vi "USBL_UA TRACKER for boat.vi"() -> ()   [LabVIEW 2017]
uses:
  <vilib>/Analysis/2dsp.llb/Decimate (single shot, DBL).vi
  <vilib>/DAQmx/read.llb/DAQmx Read (Analog 1D Wfm NChan NSamp).vi
  38e43d16-6990-4eb8-9d42-40b952a00b57.vi
  25bd1765-28c0-4687-a34a-e202199d80b9.vi
  7c68f900-8937-4c41-aeac-c7f4ae5d0ac2.vi
  eb8648f9-6bcc-41d4-a5ab-eca906629b06.vi
  bc7cbcab-f54e-4253-b3cf-52637ffe357f.vi
  b046c4bb-afd7-42e5-9fb2-1f2d57cd0f45.vi
  21d9bc29-df65-4687-956e-6793f94ae84a.vi
  72b5a707-0e99-42b5-ad5e-0d06ee7307bc.vi
  <vilib>/Array/Sort 2D Array - Pop Stack.vi
  <vilib>/Array/Sort 2D Array - Push Stack.vi
  38e43d16-6990-4eb8-9d42-40b952a00b57.vi/8e49d9bf-4fb6-4c6e-994e-0ca732c0081e.vi
  25bd1765-28c0-4687-a34a-e202199d80b9.vi/5aca4e67-a699-496d-8f3e-64a90ea83440.vi
  7c68f900-8937-4c41-aeac-c7f4ae5d0ac2.vi/c793c687-6163-4a47-8deb-c782a58a8736.vi
  eb8648f9-6bcc-41d4-a5ab-eca906629b06.vi/8c49c932-3fa2-411e-bf9f-69df11e121b8.vi
  bc7cbcab-f54e-4253-b3cf-52637ffe357f.vi/154f0d68-2825-48c0-8ee2-adf7998e7ff9.vi
  b046c4bb-afd7-42e5-9fb2-1f2d57cd0f45.vi/c2f5fb0a-7bab-41dc-aee0-b17c4b21b3df.vi
  21d9bc29-df65-4687-956e-6793f94ae84a.vi/e3f212c9-88b2-4250-9581-4cd035c99f0d.vi
  72b5a707-0e99-42b5-ad5e-0d06ee7307bc.vi/54bdf0c9-fde7-4a65-a34a-a18ed20cf916.vi
  <vilib>/Analysis/3filter.llb/FIR Filter (DBL).vi
  <vilib>/DAQmx/create/channels.llb/DAQmx Create Channel (AI-Voltage-Basic).vi
  <vilib>/DAQmx/configure/timing.llb/DAQmx Timing (Sample Clock).vi
  <vilib>/DAQmx/miscellaneous.llb/DAQmx Fill In Error Info.vi
  <vilib>/DAQmx/create/channels.llb/DAQmx Create Channel (CO-Pulse Generation-Frequency).vi
  <vilib>/DAQmx/configure/timing.llb/DAQmx Timing (Implicit).vi
  <vilib>/Analysis/NI_AALBase.lvlib
  <vilib>/Analysis/NI_AALPro.lvlib
  <vilib>/Analysis/NI_AAL_SigProc.lvlib
  <resource>/objmgr/daqmx.rc
  <vilib>/httpClient/LabVIEWHTTPClient.lvlib
panel:
  out "not detected number":i32
  out "DoA trial number":i32
  out "DoA":dbl
  out "Distance":dbl
  out "Display":bool
  out "DoA Estimation":bool
  out "Signal processing":bool
  in  "Map Format":string(combo)="roadmap"
  in  "Size X":dbl=450.0
  in  "Size Y":dbl=650.0
  in  "Zoom":sgl=16.0 format="%#.1g"
  in  "WebBrowser":refnum<k7>(container) caption="웹 브라우저"
  in  "Logitude":string="129.15510"
  in  "Latitude":string="35.17100"
  out "Scope":picture
  out "MovingAverage_Coefficient":dbl[](array[numeric])=[0.0004, 0.0004, 0.0004, 0.0004, 0.0004, 0.0004, 0.0004, 0.0004, 0.0004, 0.0004, 0.0004, 0.0004, 0.0004, 0.0004, 0.0004, 0.0004, 0.0004, 0.0004, 0.0004, 0.0004, 0.0004, 0.0004, 0.0004, 0.0004, 0.0004, 0.0004, 0.0004, 0.0004, 0.0004, 0.0004, 0.0004, 0.0004, 0.0004, 0.0004, 0.0004, 0.0004, 0.0004, 0.0004, 0.0004, 0.0004, 0.0004, 0.0004, 0.0004, 0.0004, 0.0004, 0.0004, 0.0004, 0.0004, 0.0004, 0.0004, 0.0004, 0.0004, 0.0004, 0.0004, 0.0004, 0.0004, 0.0004, 0.0004, 0.0004, 0.0004, 0.0004, 0.0004, 0.0004, 0.0004, 0.0004, 0.0004, 0.0004, 0.0004, 0.0004, 0.0004, 0.0004, 0.0004, 0.0004, 0.0004, 0.0004, 0.0004, 0.0004, 0.0004, 0.0004, 0.0004, 0.0004, 0.0004, 0.0004, 0.0004, 0.0004, 0.0004, 0.0004, 0.0004, 0.0004, 0.0004, 0.0004, 0.0004, 0.0004, 0.0004, 0.0004, 0.0004, 0.0004, 0.0004, 0.0004, 0.0004, 0.0004, 0.0004, 0.0004, 0.0004, 0.0004, 0.0004, 0.0004, 0.0004, 0.0004, 0.0004, 0.0004, 0.0004, 0.0004, 0.0004, 0.0004, 0.0004, 0.0004, 0.0004, 0.0004, 0.0004, 0.0004, 0.0004, 0.0004, 0.0004, 0.0004, 0.0004, 0.0004, 0.0004, 0.0004, 0.0004, 0.0004, 0.0004, 0.0004, 0.0004, 0.0004, 0.0004, 0.0004, 0.0004, 0.0004, 0.0004, 0.0004, 0.0004, 0.0004, 0.0004, 0.0004, 0.0004, 0.0004, 0.0004, 0.0004, 0.0004, 0.0004, 0.0004, 0.0004, 0.0004, 0.0004, 0.0004, 0.0004, 0.0004, 0.0004, 0.0004, 0.0004, 0.0004, 0.0004, 0.0004, 0.0004, 0.0004, 0.0004, 0.0004, 0.0004, 0.0004, 0.0004, 0.0004, 0.0004, 0.0004, 0.0004, 0.0004, 0.0004, 0.0004, 0.0004, 0.0004, 0.0004, 0.0004, 0.0004, 0.0004, 0.0004, 0.0004, 0.0004, 0.0004, 0.0004, 0.0004, 0.0004, 0.0004, 0.0004, 0.0004, 0.0004, 0.0004, 0.0004, 0.0004, 0.0004, 0.0004, 0.0004, 0.0004, 0.0004, 0.0004, 0.0004, 0.0004, 0.0004, 0.0004, 0.0004, 0.0004, 0.0004, 0.0004, 0.0004, 0.0004, 0.0004, 0.0004, 0.0004, 0.0004, 0.0004, 0.0004, 0.0004, 0.0004, 0.0004, 0.0004, 0.0004, 0.0004, 0.0004, 0.0004, 0.0004, 0.0004, 0.0004, 0.0004, 0.0004, 0.0004, 0.0004, 0.0004, 0.0004, 0.0004, 0.0004, 0.0004, 0.0004, 0.0004, 0.0004, 0.0004, 0.0004, 0.0004, 0.0004, 0.0004, 0.0004, 0.0004, 0.0004, 0.0004, 0.0004, 0.0004, 0.0004, 0.0004, 0.0004, 0.0004, 0.0004, 0.0004, 0.0004, 0.0004, 0.0004, 0.0004, 0.0004, 0.0004, 0.0004, 0.0004, 0.0004, 0.0004, 0.0004, 0.0004, 0.0004, 0.0004, 0.0004, 0.0004, 0.0004, 0.0004, 0.0004, 0.0004, 0.0004, 0.0004, 0.0004, 0.0004, 0.0004, 0.0004, 0.0004, 0.0004, 0.0004, 0.0004, 0.0004, 0.0004, 0.0004, 0.0004, 0.0004, 0.0004, 0.0004, 0.0004, 0.0004, 0.0004, 0.0004, 0.0004, 0.0004, 0.0004, 0.0004, 0.0004, 0.0004, 0.0004, 0.0004, 0.0004, 0.0004, 0.0004, 0.0004, 0.0004, 0.0004, 0.0004, 0.0004, 0.0004, 0.0004, 0.0004, 0.0004, 0.0004, 0.0004, 0.0004, 0.0004, 0.0004, 0.0004, 0.0004, 0.0004, 0.0004, 0.0004, 0.0004, 0.0004, 0.0004, 0.0004, 0.0004, 0.0004, 0.0004, 0.0004, 0.0004, 0.0004, 0.0004, 0.0004, 0.0004, 0.0004, 0.0004, 0.0004, 0.0004, 0.0004, 0.0004, 0.0004, 0.0004, 0.0004, 0.0004, 0.0004, 0.0004, 0.0004, 0.0004, 0.0004, 0.0004, 0.0004, 0.0004, 0.0004, 0.0004, 0.0004, 0.0004, 0.0004, 0.0004, 0.0004, 0.0004, 0.0004, 0.0004, 0.0004, 0.0004, 0.0004, 0.0004, 0.0004, 0.0004, 0.0004, 0.0004, 0.0004, 0.0004, 0.0004, 0.0004, 0.0004, 0.0004, 0.0004, 0.0004, 0.0004, 0.0004, 0.0004, 0.0004, 0.0004, 0.0004, 0.0004, 0.0004, 0.0004, 0.0004, 0.0004, 0.0004, 0.0004, 0.0004, 0.0004, 0.0004, 0.0004, 0.0004, 0.0004, 0.0004, 0.0004, 0.0004, 0.0004, 0.0004, 0.0004, 0.0004, 0.0004, 0.0004, 0.0004, 0.0004, 0.0004, 0.0004, 0.0004, 0.0004, 0.0004, 0.0004, 0.0004, 0.0004, 0.0004, 0.0004, 0.0004, 0.0004, 0.0004, 0.0004, 0.0004, 0.0004, 0.0004, 0.0004, 0.0004, 0.0004, 0.0004, 0.0004, 0.0004, 0.0004, 0.0004, 0.0004, 0.0004, 0.0004, 0.0004, 0.0004, 0.0004, 0.0004, 0.0004, 0.0004, 0.0004, 0.0004, 0.0004, 0.0004, 0.0004, 0.0004, 0.0004, 0.0004, 0.0004, 0.0004, 0.0004, 0.0004, 0.0004, 0.0004, 0.0004, 0.0004, 0.0004, 0.0004, 0.0004, 0.0004, 0.0004, 0.0004, 0.0004, 0.0004, 0.0004, 0.0004, 0.0004, 0.0004, 0.0004, 0.0004, 0.0004, 0.0004, 0.0004, 0.0004, 0.0004, 0.0004, 0.0004, 0.0004, 0.0004, 0.0004, 0.0004, 0.0004, 0.0004, 0.0004, 0.0004, 0.0004, 0.0004, 0.0004, 0.0004, 0.0004, 0.0004, 0.0004, 0.0004, 0.0004, 0.0004, 0.0004, 0.0004, 0.0004, 0.0004, 0.0004, 0.0004, 0.0004, 0.0004, 0.0004, 0.0004, 0.0004, 0.0004, 0.0004, 0.0004, 0.0004, 0.0004, 0.0004, 0.0004, 0.0004, 0.0004, 0.0004, 0.0004, 0.0004, 0.0004, 0.0004, 0.0004, 0.0004, 0.0004, 0.0004, 0.0004, 0.0004, 0.0004, 0.0004, 0.0004, 0.0004, 0.0004, 0.0004, 0.0004, 0.0004, 0.0004, 0.0004, 0.0004, 0.0004, 0.0004, 0.0004, 0.0004, 0.0004, 0.0004, 0.0004, 0.0004, 0.0004, 0.0004, 0.0004, 0.0004, 0.0004, 0.0004, 0.0004, 0.0004, 0.0004, 0.0004, 0.0004, 0.0004, 0.0004, 0.0004, 0.0004, 0.0004, 0.0004, 0.0004, 0.0004, 0.0004, 0.0004, 0.0004, 0.0004, 0.0004, 0.0004, 0.0004, 0.0004, 0.0004, 0.0004, 0.0004, 0.0004, 0.0004, 0.0004, 0.0004, 0.0004, 0.0004, 0.0004, 0.0004, 0.0004, 0.0004, 0.0004, 0.0004, 0.0004, 0.0004, 0.0004, 0.0004, 0.0004, 0.0004, 0.0004, 0.0004, 0.0004, 0.0004, 0.0004, 0.0004, 0.0004, 0.0004, 0.0004, 0.0004, 0.0004, 0.0004, 0.0004, 0.0004, 0.0004, 0.0004, 0.0004, 0.0004, 0.0004, 0.0004, 0.0004, 0.0004, 0.0004, 0.0004, 0.0004, 0.0004, 0.0004, 0.0004, 0.0004, 0.0004, 0.0004, 0.0004, 0.0004, 0.0004, 0.0004, 0.0004, 0.0004, 0.0004, 0.0004, 0.0004, 0.0004, 0.0004, 0.0004, 0.0004, 0.0004, 0.0004, 0.0004, 0.0004, 0.0004, 0.0004, 0.0004, 0.0004, 0.0004, 0.0004, 0.0004, 0.0004, 0.0004, 0.0004, 0.0004, 0.0004, 0.0004, 0.0004, 0.0004, 0.0004, 0.0004, 0.0004, 0.0004, 0.0004, 0.0004, 0.0004, 0.0004, 0.0004, 0.0004, 0.0004, 0.0004, 0.0004, 0.0004, 0.0004, 0.0004, 0.0004, 0.0004, 0.0004, 0.0004, 0.0004, 0.0004, 0.0004, 0.0004, 0.0004, 0.0004, 0.0004, 0.0004, 0.0004, 0.0004, 0.0004, 0.0004, 0.0004, 0.0004, 0.0004, 0.0004, 0.0004, 0.0004, 0.0004, 0.0004, 0.0004, 0.0004, 0.0004, 0.0004, 0.0004, 0.0004, 0.0004, 0.0004, 0.0004, 0.0004, 0.0004, 0.0004, 0.0004, 0.0004, 0.0004, 0.0004, 0.0004, 0.0004, 0.0004, 0.0004, 0.0004, 0.0004, 0.0004, 0.0004, 0.0004, 0.0004, 0.0004, 0.0004, 0.0004, 0.0004, 0.0004, 0.0004, 0.0004, 0.0004, 0.0004, 0.0004, 0.0004, 0.0004, 0.0004, 0.0004, 0.0004, 0.0004, 0.0004, 0.0004, 0.0004, 0.0004, 0.0004, 0.0004, 0.0004, 0.0004, 0.0004, 0.0004, 0.0004, 0.0004, 0.0004, 0.0004, 0.0004, 0.0004, 0.0004, 0.0004, 0.0004, 0.0004, 0.0004, 0.0004, 0.0004, 0.0004, 0.0004, 0.0004, 0.0004, 0.0004, 0.0004, 0.0004, 0.0004, 0.0004, 0.0004, 0.0004, 0.0004, 0.0004, 0.0004, 0.0004, 0.0004, 0.0004, 0.0004, 0.0004, 0.0004, 0.0004, 0.0004, 0.0004, 0.0004, 0.0004, 0.0004, 0.0004, 0.0004, 0.0004, 0.0004, 0.0004, 0.0004, 0.0004, 0.0004, 0.0004, 0.0004, 0.0004, 0.0004, 0.0004, 0.0004, 0.0004, 0.0004, 0.0004, 0.0004, 0.0004, 0.0004, 0.0004, 0.0004, 0.0004, 0.0004, 0.0004, 0.0004, 0.0004, 0.0004, 0.0004, 0.0004, 0.0004, 0.0004, 0.0004, 0.0004, 0.0004, 0.0004, 0.0004, 0.0004, 0.0004, 0.0004, 0.0004, 0.0004, 0.0004, 0.0004, 0.0004, 0.0004, 0.0004, 0.0004, 0.0004, 0.0004, 0.0004, 0.0004, 0.0004, 0.0004, 0.0004, 0.0004, 0.0004, 0.0004, 0.0004, 0.0004, 0.0004, 0.0004, 0.0004, 0.0004, 0.0004, 0.0004, 0.0004, 0.0004, 0.0004, 0.0004, 0.0004, 0.0004, 0.0004, 0.0004, 0.0004, 0.0004, 0.0004, 0.0004, 0.0004, 0.0004, 0.0004, 0.0004, 0.0004, 0.0004, 0.0004, 0.0004, 0.0004, 0.0004, 0.0004, 0.0004, 0.0004, 0.0004, 0.0004, 0.0004, 0.0004, 0.0004, 0.0004, 0.0004, 0.0004, 0.0004, 0.0004, 0.0004, 0.0004, 0.0004, 0.0004, 0.0004, 0.0004, 0.0004, 0.0004, 0.0004, 0.0004, 0.0004, 0.0004, 0.0004, 0.0004, 0.0004, 0.0004, 0.0004, 0.0004, 0.0004, 0.0004, 0.0004, 0.0004, 0.0004, 0.0004, 0.0004, 0.0004, 0.0004, 0.0004, 0.0004, 0.0004, 0.0004, 0.0004, 0.0004, 0.0004, 0.0004, 0.0004, 0.0004, 0.0004, 0.0004, 0.0004, 0.0004, 0.0004, 0.0004, 0.0004, 0.0004, 0.0004, 0.0004, 0.0004, 0.0004, 0.0004, 0.0004, 0.0004, 0.0004, 0.0004, 0.0004, 0.0004, 0.0004, 0.0004, 0.0004, 0.0004, 0.0004, 0.0004, 0.0004, 0.0004, 0.0004, 0.0004, 0.0004, 0.0004, 0.0004, 0.0004, 0.0004, 0.0004, 0.0004, 0.0004, 0.0004, 0.0004, 0.0004, 0.0004, 0.0004, 0.0004, 0.0004, 0.0004, 0.0004, 0.0004, 0.0004, 0.0004, 0.0004, 0.0004, 0.0004, 0.0004, 0.0004, 0.0004, 0.0004, 0.0004, 0.0004, 0.0004, 0.0004, 0.0004, 0.0004, 0.0004, 0.0004, 0.0004, 0.0004, 0.0004, 0.0004, 0.0004, 0.0004, 0.0004, 0.0004, 0.0004, 0.0004, 0.0004, 0.0004, 0.0004, 0.0004, 0.0004, 0.0004, 0.0004, 0.0004, 0.0004, 0.0004, 0.0004, 0.0004, 0.0004, 0.0004, 0.0004, 0.0004, 0.0004, 0.0004, 0.0004, 0.0004, 0.0004, 0.0004, 0.0004, 0.0004, 0.0004, 0.0004, 0.0004, 0.0004, 0.0004, 0.0004, 0.0004, 0.0004, 0.0004, 0.0004, 0.0004, 0.0004, 0.0004, 0.0004, 0.0004, 0.0004, 0.0004, 0.0004, 0.0004, 0.0004, 0.0004, 0.0004, 0.0004, 0.0004, 0.0004, 0.0004, 0.0004, 0.0004, 0.0004, 0.0004, 0.0004, 0.0004, 0.0004, 0.0004, 0.0004, 0.0004, 0.0004, 0.0004, 0.0004, 0.0004, 0.0004, 0.0004, 0.0004, 0.0004, 0.0004, 0.0004, 0.0004, 0.0004, 0.0004, 0.0004, 0.0004, 0.0004, 0.0004, 0.0004, 0.0004, 0.0004, 0.0004, 0.0004, 0.0004, 0.0004, 0.0004, 0.0004, 0.0004, 0.0004, 0.0004, 0.0004, 0.0004, 0.0004, 0.0004, 0.0004, 0.0004, 0.0004, 0.0004, 0.0004, 0.0004, 0.0004, 0.0004, 0.0004, 0.0004, 0.0004, 0.0004, 0.0004, 0.0004, 0.0004, 0.0004, 0.0004, 0.0004, 0.0004, 0.0004, 0.0004, 0.0004, 0.0004, 0.0004, 0.0004, 0.0004, 0.0004, 0.0004, 0.0004, 0.0004, 0.0004, 0.0004, 0.0004, 0.0004, 0.0004, 0.0004, 0.0004, 0.0004, 0.0004, 0.0004, 0.0004, 0.0004, 0.0004, 0.0004, 0.0004, 0.0004, 0.0004, 0.0004, 0.0004, 0.0004, 0.0004, 0.0004, 0.0004, 0.0004, 0.0004, 0.0004, 0.0004, 0.0004, 0.0004, 0.0004, 0.0004, 0.0004, 0.0004, 0.0004, 0.0004, 0.0004, 0.0004, 0.0004, 0.0004, 0.0004, 0.0004, 0.0004, 0.0004, 0.0004, 0.0004, 0.0004, 0.0004, 0.0004, 0.0004, 0.0004, 0.0004, 0.0004, 0.0004, 0.0004, 0.0004, 0.0004, 0.0004, 0.0004, 0.0004, 0.0004, 0.0004, 0.0004, 0.0004, 0.0004, 0.0004, 0.0004, 0.0004, 0.0004, 0.0004, 0.0004, 0.0004, 0.0004, 0.0004, 0.0004, 0.0004, 0.0004, 0.0004, 0.0004, 0.0004, 0.0004, 0.0004, 0.0004, 0.0004, 0.0004, 0.0004, 0.0004, 0.0004, 0.0004, 0.0004, 0.0004, 0.0004, 0.0004, 0.0004, 0.0004, 0.0004, 0.0004, 0.0004, 0.0004, 0.0004, 0.0004, 0.0004, 0.0004, 0.0004, 0.0004, 0.0004, 0.0004, 0.0004, 0.0004, 0.0004, 0.0004, 0.0004, 0.0004, 0.0004, 0.0004, 0.0004, 0.0004, 0.0004, 0.0004, 0.0004, 0.0004, 0.0004, 0.0004, 0.0004, 0.0004, 0.0004, 0.0004, 0.0004, 0.0004, 0.0004, 0.0004, 0.0004, 0.0004, 0.0004, 0.0004, 0.0004, 0.0004, 0.0004, 0.0004, 0.0004, 0.0004, 0.0004, 0.0004, 0.0004, 0.0004, 0.0004, 0.0004, 0.0004, 0.0004, 0.0004, 0.0004, 0.0004, 0.0004, 0.0004, 0.0004, 0.0004, 0.0004, 0.0004, 0.0004, 0.0004, 0.0004, 0.0004, 0.0004, 0.0004, 0.0004, 0.0004, 0.0004, 0.0004, 0.0004, 0.0004, 0.0004, 0.0004, 0.0004, 0.0004, 0.0004, 0.0004, 0.0004, 0.0004, 0.0004, 0.0004, 0.0004, 0.0004, 0.0004, 0.0004, 0.0004, 0.0004, 0.0004, 0.0004, 0.0004, 0.0004, 0.0004, 0.0004, 0.0004, 0.0004, 0.0004, 0.0004, 0.0004, 0.0004, 0.0004, 0.0004, 0.0004, 0.0004, 0.0004, 0.0004, 0.0004, 0.0004, 0.0004, 0.0004, 0.0004, 0.0004, 0.0004, 0.0004, 0.0004, 0.0004, 0.0004, 0.0004, 0.0004, 0.0004, 0.0004, 0.0004, 0.0004, 0.0004, 0.0004, 0.0004, 0.0004, 0.0004, 0.0004, 0.0004, 0.0004, 0.0004, 0.0004, 0.0004, 0.0004, 0.0004, 0.0004, 0.0004, 0.0004, 0.0004, 0.0004, 0.0004, 0.0004, 0.0004, 0.0004, 0.0004, 0.0004, 0.0004, 0.0004, 0.0004, 0.0004, 0.0004, 0.0004, 0.0004, 0.0004, 0.0004, 0.0004, 0.0004, 0.0004, 0.0004, 0.0004, 0.0004, 0.0004, 0.0004, 0.0004, 0.0004, 0.0004, 0.0004, 0.0004, 0.0004, 0.0004, 0.0004, 0.0004, 0.0004, 0.0004, 0.0004, 0.0004, 0.0004, 0.0004, 0.0004, 0.0004, 0.0004, 0.0004, 0.0004, 0.0004, 0.0004, 0.0004, 0.0004, 0.0004, 0.0004, 0.0004, 0.0004, 0.0004, 0.0004, 0.0004, 0.0004, 0.0004, 0.0004, 0.0004, 0.0004, 0.0004, 0.0004, 0.0004, 0.0004, 0.0004, 0.0004, 0.0004, 0.0004, 0.0004, 0.0004, 0.0004, 0.0004, 0.0004, 0.0004, 0.0004, 0.0004, 0.0004, 0.0004, 0.0004, 0.0004, 0.0004, 0.0004, 0.0004, 0.0004, 0.0004, 0.0004, 0.0004, 0.0004, 0.0004, 0.0004, 0.0004, 0.0004, 0.0004, 0.0004, 0.0004, 0.0004, 0.0004, 0.0004, 0.0004, 0.0004, 0.0004, 0.0004, 0.0004, 0.0004, 0.0004, 0.0004, 0.0004, 0.0004, 0.0004, 0.0004, 0.0004, 0.0004, 0.0004, 0.0004, 0.0004, 0.0004, 0.0004, 0.0004, 0.0004, 0.0004, 0.0004, 0.0004, 0.0004, 0.0004, 0.0004, 0.0004, 0.0004, 0.0004, 0.0004, 0.0004, 0.0004, 0.0004, 0.0004, 0.0004, 0.0004, 0.0004, 0.0004, 0.0004, 0.0004, 0.0004, 0.0004, 0.0004, 0.0004, 0.0004, 0.0004, 0.0004, 0.0004, 0.0004, 0.0004, 0.0004, 0.0004, 0.0004, 0.0004, 0.0004, 0.0004, 0.0004, 0.0004, 0.0004, 0.0004, 0.0004, 0.0004, 0.0004, 0.0004, 0.0004, 0.0004, 0.0004, 0.0004, 0.0004, 0.0004, 0.0004, 0.0004, 0.0004, 0.0004, 0.0004, 0.0004, 0.0004, 0.0004, 0.0004, 0.0004, 0.0004, 0.0004, 0.0004, 0.0004, 0.0004, 0.0004, 0.0004, 0.0004, 0.0004, 0.0004, 0.0004, 0.0004, 0.0004, 0.0004, 0.0004, 0.0004, 0.0004, 0.0004, 0.0004, 0.0004, 0.0004, 0.0004, 0.0004, 0.0004, 0.0004, 0.0004, 0.0004, 0.0004, 0.0004, 0.0004, 0.0004, 0.0004, 0.0004, 0.0004, 0.0004, 0.0004, 0.0004, 0.0004, 0.0004, 0.0004, 0.0004, 0.0004, 0.0004, 0.0004, 0.0004, 0.0004, 0.0004, 0.0004, 0.0004, 0.0004, 0.0004, 0.0004, 0.0004, 0.0004, 0.0004, 0.0004, 0.0004, 0.0004, 0.0004, 0.0004, 0.0004, 0.0004, 0.0004, 0.0004, 0.0004, 0.0004, 0.0004, 0.0004, 0.0004, 0.0004, 0.0004, 0.0004, 0.0004, 0.0004, 0.0004, 0.0004, 0.0004, 0.0004, 0.0004, 0.0004, 0.0004, 0.0004, 0.0004, 0.0004, 0.0004, 0.0004, 0.0004, 0.0004, 0.0004, 0.0004, 0.0004, 0.0004, 0.0004, 0.0004, 0.0004, 0.0004, 0.0004, 0.0004, 0.0004, 0.0004, 0.0004, 0.0004, 0.0004, 0.0004, 0.0004, 0.0004, 0.0004, 0.0004, 0.0004, 0.0004, 0.0004, 0.0004, 0.0004, 0.0004, 0.0004, 0.0004, 0.0004, 0.0004, 0.0004, 0.0004, 0.0004, 0.0004, 0.0004, 0.0004, 0.0004, 0.0004, 0.0004, 0.0004, 0.0004, 0.0004, 0.0004, 0.0004, 0.0004, 0.0004, 0.0004, 0.0004, 0.0004, 0.0004, 0.0004, 0.0004, 0.0004, 0.0004, 0.0004, 0.0004, 0.0004, 0.0004, 0.0004, 0.0004, 0.0004, 0.0004, 0.0004, 0.0004, 0.0004, 0.0004, 0.0004, 0.0004, 0.0004, 0.0004, 0.0004, 0.0004, 0.0004, 0.0004, 0.0004, 0.0004, 0.0004, 0.0004, 0.0004, 0.0004, 0.0004, 0.0004, 0.0004, 0.0004, 0.0004, 0.0004, 0.0004, 0.0004, 0.0004, 0.0004, 0.0004, 0.0004, 0.0004, 0.0004, 0.0004, 0.0004, 0.0004, 0.0004, 0.0004, 0.0004, 0.0004, 0.0004, 0.0004, 0.0004, 0.0004, 0.0004, 0.0004, 0.0004, 0.0004, 0.0004, 0.0004, 0.0004, 0.0004, 0.0004, 0.0004, 0.0004, 0.0004, 0.0004, 0.0004, 0.0004, 0.0004, 0.0004, 0.0004, 0.0004, 0.0004, 0.0004, 0.0004, 0.0004, 0.0004, 0.0004, 0.0004, 0.0004, 0.0004, 0.0004, 0.0004, 0.0004, 0.0004, 0.0004, 0.0004, 0.0004, 0.0004, 0.0004, 0.0004, 0.0004, 0.0004, 0.0004, 0.0004, 0.0004, 0.0004, 0.0004, 0.0004, 0.0004, 0.0004, 0.0004, 0.0004, 0.0004, 0.0004, 0.0004, 0.0004, 0.0004, 0.0004, 0.0004, 0.0004, 0.0004, 0.0004, 0.0004, 0.0004, 0.0004, 0.0004, 0.0004, 0.0004, 0.0004, 0.0004, 0.0004, 0.0004, 0.0004, 0.0004, 0.0004, 0.0004, 0.0004, 0.0004, 0.0004, 0.0004, 0.0004, 0.0004, 0.0004, 0.0004, 0.0004, 0.0004, 0.0004, 0.0004, 0.0004, 0.0004, 0.0004, 0.0004, 0.0004, 0.0004, 0.0004, 0.0004, 0.0004, 0.0004, 0.0004, 0.0004, 0.0004, 0.0004, 0.0004, 0.0004, 0.0004, 0.0004, 0.0004, 0.0004, 0.0004, 0.0004, 0.0004, 0.0004, 0.0004, 0.0004, 0.0004, 0.0004, 0.0004, 0.0004, 0.0004, 0.0004, 0.0004, 0.0004, 0.0004, 0.0004, 0.0004, 0.0004, 0.0004, 0.0004, 0.0004, 0.0004, 0.0004, 0.0004, 0.0004, 0.0004, 0.0004, 0.0004, 0.0004, 0.0004, 0.0004, 0.0004, 0.0004, 0.0004, 0.0004, 0.0004, 0.0004, 0.0004, 0.0004, 0.0004, 0.0004, 0.0004, 0.0004, 0.0004, 0.0004, 0.0004, 0.0004, 0.0004, 0.0004, 0.0004, 0.0004, 0.0004, 0.0004, 0.0004, 0.0004, 0.0004, 0.0004, 0.0004, 0.0004, 0.0004, 0.0004, 0.0004, 0.0004, 0.0004, 0.0004, 0.0004, 0.0004, 0.0004, 0.0004, 0.0004, 0.0004, 0.0004, 0.0004, 0.0004, 0.0004, 0.0004, 0.0004, 0.0004, 0.0004, 0.0004, 0.0004, 0.0004, 0.0004, 0.0004, 0.0004, 0.0004, 0.0004, 0.0004, 0.0004, 0.0004, 0.0004, 0.0004, 0.0004, 0.0004, 0.0004, 0.0004, 0.0004, 0.0004, 0.0004, 0.0004, 0.0004, 0.0004, 0.0004, 0.0004, 0.0004, 0.0004, 0.0004, 0.0004, 0.0004, 0.0004, 0.0004, 0.0004, 0.0004, 0.0004, 0.0004, 0.0004, 0.0004, 0.0004, 0.0004, 0.0004, 0.0004, 0.0004, 0.0004, 0.0004, 0.0004, 0.0004, 0.0004, 0.0004, 0.0004, 0.0004, 0.0004, 0.0004, 0.0004, 0.0004, 0.0004, 0.0004, 0.0004, 0.0004, 0.0004, 0.0004, 0.0004, 0.0004, 0.0004, 0.0004, 0.0004, 0.0004, 0.0004, 0.0004, 0.0004, 0.0004, 0.0004, 0.0004, 0.0004, 0.0004, 0.0004, 0.0004, 0.0004, 0.0004, 0.0004, 0.0004, 0.0004, 0.0004, 0.0004, 0.0004, 0.0004, 0.0004, 0.0004, 0.0004, 0.0004, 0.0004, 0.0004, 0.0004, 0.0004, 0.0004, 0.0004, 0.0004, 0.0004, 0.0004, 0.0004, 0.0004, 0.0004, 0.0004, 0.0004, 0.0004, 0.0004, 0.0004, 0.0004, 0.0004, 0.0004, 0.0004, 0.0004, 0.0004, 0.0004, 0.0004, 0.0004, 0.0004, 0.0004, 0.0004, 0.0004, 0.0004, 0.0004, 0.0004, 0.0004, 0.0004, 0.0004, 0.0004, 0.0004, 0.0004, 0.0004, 0.0004, 0.0004, 0.0004, 0.0004, 0.0004, 0.0004, 0.0004, 0.0004, 0.0004, 0.0004, 0.0004, 0.0004, 0.0004, 0.0004, 0.0004, 0.0004, 0.0004, 0.0004, 0.0004, 0.0004, 0.0004, 0.0004, 0.0004, 0.0004, 0.0004, 0.0004, 0.0004, 0.0004, 0.0004, 0.0004, 0.0004, 0.0004, 0.0004, 0.0004, 0.0004, 0.0004, 0.0004, 0.0004, 0.0004, 0.0004, 0.0004, 0.0004, 0.0004, 0.0004, 0.0004, 0.0004, 0.0004, 0.0004, 0.0004, 0.0004, 0.0004, 0.0004, 0.0004, 0.0004, 0.0004, 0.0004, 0.0004, 0.0004, 0.0004, 0.0004, 0.0004, 0.0004, 0.0004, 0.0004, 0.0004, 0.0004, 0.0004, 0.0004, 0.0004, 0.0004, 0.0004, 0.0004, 0.0004, 0.0004, 0.0004, 0.0004, 0.0004, 0.0004, 0.0004, 0.0004, 0.0004, 0.0004, 0.0004, 0.0004, 0.0004, 0.0004, 0.0004, 0.0004, 0.0004, 0.0004, 0.0004, 0.0004, 0.0004, 0.0004, 0.0004, 0.0004, 0.0004, 0.0004, 0.0004, 0.0004, 0.0004, 0.0004, 0.0004, 0.0004, 0.0004, 0.0004, 0.0004, 0.0004, 0.0004, 0.0004, 0.0004, 0.0004, 0.0004, 0.0004, 0.0004, 0.0004, 0.0004, 0.0004, 0.0004, 0.0004, 0.0004, 0.0004, 0.0004, 0.0004, 0.0004, 0.0004, 0.0004, 0.0004, 0.0004, 0.0004, 0.0004, 0.0004, 0.0004, 0.0004, 0.0004, 0.0004, 0.0004, 0.0004, 0.0004, 0.0004, 0.0004, 0.0004, 0.0004, 0.0004, 0.0004, 0.0004, 0.0004, 0.0004, 0.0004, 0.0004, 0.0004, 0.0004, 0.0004, 0.0004, 0.0004, 0.0004, 0.0004, 0.0004, 0.0004, 0.0004, 0.0004, 0.0004, 0.0004, 0.0004, 0.0004, 0.0004, 0.0004, 0.0004, 0.0004, 0.0004, 0.0004, 0.0004, 0.0004, 0.0004, 0.0004, 0.0004, 0.0004, 0.0004, 0.0004, 0.0004, 0.0004, 0.0004, 0.0004, 0.0004, 0.0004, 0.0004, 0.0004, 0.0004, 0.0004, 0.0004, 0.0004, 0.0004, 0.0004, 0.0004, 0.0004, 0.0004, 0.0004, 0.0004, 0.0004, 0.0004, 0.0004, 0.0004, 0.0004, 0.0004, 0.0004, 0.0004, 0.0004, 0.0004, 0.0004, 0.0004, 0.0004, 0.0004, 0.0004, 0.0004, 0.0004, 0.0004, 0.0004, 0.0004, 0.0004, 0.0004, 0.0004, 0.0004, 0.0004, 0.0004, 0.0004, 0.0004, 0.0004, 0.0004, 0.0004, 0.0004, 0.0004, 0.0004, 0.0004, 0.0004, 0.0004, 0.0004, 0.0004, 0.0004, 0.0004, 0.0004, 0.0004, 0.0004, 0.0004, 0.0004, 0.0004, 0.0004, 0.0004, 0.0004, 0.0004, 0.0004, 0.0004, 0.0004, 0.0004, 0.0004, 0.0004, 0.0004, 0.0004, 0.0004, 0.0004, 0.0004, 0.0004, 0.0004, 0.0004, 0.0004, 0.0004, 0.0004, 0.0004, 0.0004, 0.0004, 0.0004, 0.0004, 0.0004, 0.0004, 0.0004, 0.0004, 0.0004, 0.0004, 0.0004, 0.0004, 0.0004, 0.0004, 0.0004, 0.0004, 0.0004, 0.0004, 0.0004, 0.0004, 0.0004, 0.0004, 0.0004, 0.0004, 0.0004, 0.0004, 0.0004, 0.0004, 0.0004, 0.0004, 0.0004, 0.0004, 0.0004, 0.0004, 0.0004, 0.0004, 0.0004, 0.0004, 0.0004, 0.0004, 0.0004, 0.0004, 0.0004, 0.0004, 0.0004, 0.0004, 0.0004, 0.0004, 0.0004, 0.0004, 0.0004, 0.0004, 0.0004, 0.0004, 0.0004, 0.0004, 0.0004, 0.0004, 0.0004, 0.0004, 0.0004, 0.0004, 0.0004, 0.0004, 0.0004, 0.0004, 0.0004, 0.0004, 0.0004, 0.0004, 0.0004, 0.0004, 0.0004, 0.0004, 0.0004, 0.0004, 0.0004, 0.0004, 0.0004, 0.0004, 0.0004, 0.0004, 0.0004, 0.0004, 0.0004, 0.0004, 0.0004, 0.0004, 0.0004, 0.0004, 0.0004, 0.0004, 0.0004, 0.0004, 0.0004, 0.0004, 0.0004, 0.0004, 0.0004, 0.0004, 0.0004, 0.0004, 0.0004, 0.0004, 0.0004, 0.0004, 0.0004, 0.0004, 0.0004, 0.0004, 0.0004, 0.0004, 0.0004, 0.0004, 0.0004, 0.0004, 0.0004, 0.0004, 0.0004, 0.0004, 0.0004, 0.0004, 0.0004, 0.0004, 0.0004, 0.0004, 0.0004, 0.0004, 0.0004, 0.0004, 0.0004, 0.0004, 0.0004, 0.0004, 0.0004, 0.0004, 0.0004, 0.0004, 0.0004, 0.0004, 0.0004, 0.0004, 0.0004, 0.0004, 0.0004, 0.0004, 0.0004, 0.0004, 0.0004, 0.0004, 0.0004, 0.0004, 0.0004, 0.0004, 0.0004, 0.0004, 0.0004, 0.0004, 0.0004, 0.0004, 0.0004, 0.0004, 0.0004, 0.0004, 0.0004, 0.0004, 0.0004, 0.0004, 0.0004, 0.0004, 0.0004, 0.0004, 0.0004, 0.0004, 0.0004]
  out "Coefficient2_bit1":dbl[](array[numeric])
  out "Coefficient2_bit0":dbl[](array[numeric])
  in  "Start frequency(Hz) 2":dbl=30000.0 format="%#_6p"
  in  "Stop frequency(Hz) 2":dbl=34000.0 format="%#_6p"
  in  "Number of sample 2":i32=20000
  in  "Sampling freuqncy(Hz) 2":dbl=100000.0 format="%#_6p"
  out "Target code":dbl[](array[numeric])=[0.0, 1.0, 1.0, 1.0, 0.0, 0.0, 1.0, 0.0]
  in  "Number of pulse":i32=160
  in  "Output terminal":tag="/Dev4/PFI0"
  in  "Frequency(Hz)":dbl=32000.0 format="%.6f"
  in  "Cycle share":dbl=0.5 format="%.6f"
  in  "Counter":tag="Dev4/ctr0"
  out "Detect":bool
  in  "User number":i32=12
  in  "Start frequency(Hz)":dbl format="%#_6p"
  in  "Stop frequency(Hz)":dbl=4000.0 format="%#_6p"
  in  "Symbol length(sec)":dbl=0.128 format="%#_6p"
  in  "Number of sample":i32=38400
  in  "Sampling freuqncy(Hz)":dbl=192000.0 format="%#_6p"
  in  "Physical channel":tag="Dev4/ai0:7" caption="Physical Channel"
  in  "Device":tag="Dev4"
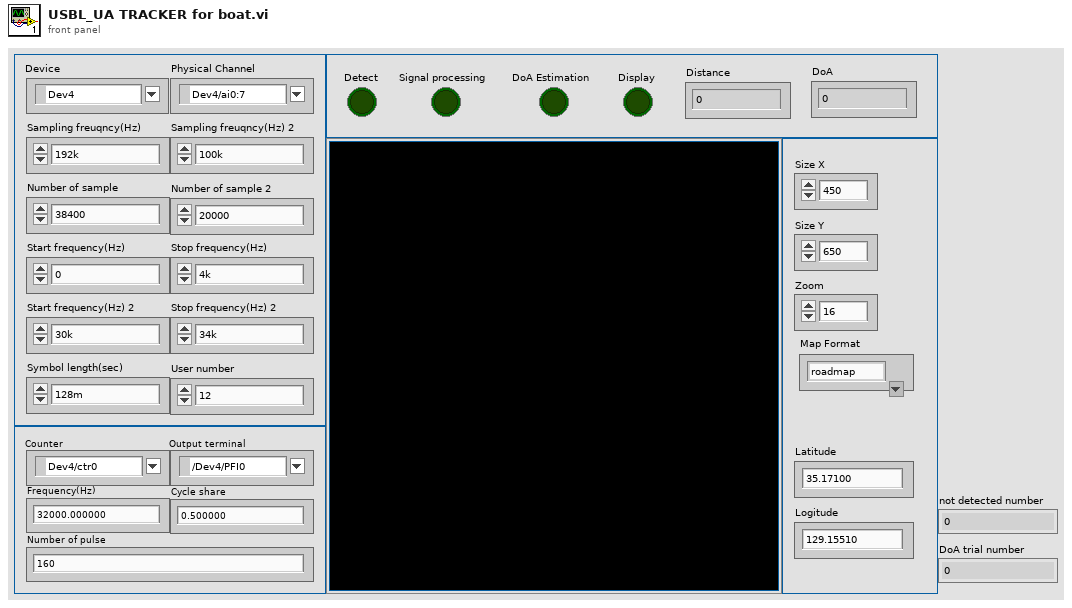
[diagram p1: front panel]
types:
  T1 = cluster{"maximum":dbl, "minimum":dbl, "clip to min":bool, "log?(F)":bool, "grid color":u32, "plot color":u32, "fmt and prec":cluster{"format":enum8{"Decimal", "Scientific", "Engineering", "Binary", "Octal", "Hex"}, "precision":u8}, "visible section":u16}
  T2 = cluster{"Marker":string, "Path":string, "Markers Coordinates":string[][]}
  T3 = typedef "LabVIEWHTTPClient.lvlib/ClientHandle.ctl" = refnum<k1>
  T4 = typedef "imagedata.ctl" = cluster{"image type":i32, "image depth":i32, "image":u8[], "mask":u8[], "colors":u32[], "Rectangle":cluster{"left":i16, "top":i16, "right":i16, "bottom":i16}}
  T5 = typedef "LVBoundsTypeDef.ctl" = cluster{"Width":u32, "Height":u32}
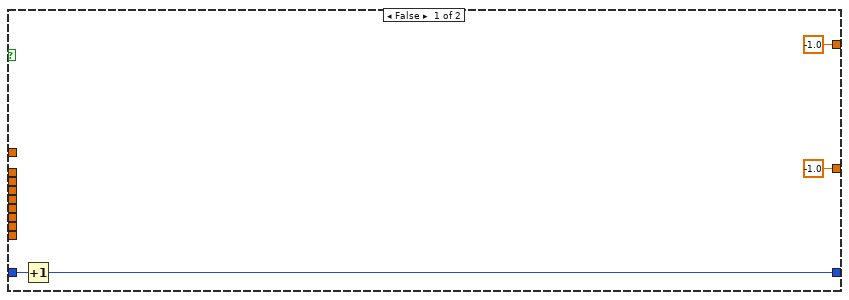
[diagram p10: hidden frame]
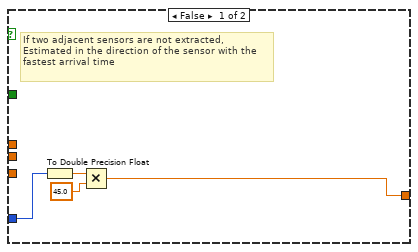
[diagram p11: hidden frame]
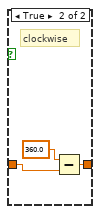
[diagram p12: hidden frame]
diagram:
  n1 = flat-sequence {
    tunnel: ["Number of sample"] -> w12
    tunnel: [w48] -> w11
    tunnel: ["Sampling freuqncy(Hz)"] -> w10
    tunnel: ["Physical channel"] -> w9
    tunnel: ["Device"] -> w8
    tunnel: [w44] -> w7
    tunnel: [w40] -> w6
    tunnel: [w39] -> w5
    tunnel: [w35] -> w4
    tunnel: [w31] -> w3
    tunnel: [10.0 ("값")] -> w2
    tunnel: [w23] -> w1
    tunnel: w12 -> [w62]
    tunnel: w11 -> [w61]
    tunnel: w10 -> [w60]
    tunnel: w9 -> [w59]
    tunnel: w8 -> [w58]
    tunnel: w7 -> [w57]
    tunnel: w6 -> [w56]
    tunnel: w5 -> [w55]
    tunnel: w4 -> [w54]
    tunnel: w3 -> [w53]
    tunnel: w2 -> [w52]
    tunnel: w1 -> [w51]
    frame #0 {
      w16 = 2500 ("차원 크기")
      w32 = 160 ("차원 크기")
      w44 = 12 ("Divide by")
      w48 = 10123 items=["유한 샘플"=10178, "연속 샘플"=10123, "하드웨어 타이밍에 의한 단일 포인트"=12522] ("sample mode")
      # "Processing parameter for mapping"
      # "Moving average window size"
      # "DAQ device setting for mapping"
      # "Signal gen. (Counter)"
      # "Target code"
      # "EOF"
      # "SOF"
      # "Processing parameter"
      # "Freqeuncy 2"
      # "Freqeuncy 1"
      # "Symbol length"
      # "Moving average window size"
      # "Threshold Margin"
      # "DAQ device setting"
      # "Device"
      # "Physical channel"
      # "Sampling frequency"
      # "Sample mode"
      # "Number of samples per channel"
      n2 = To Double Precision Float(number=w44) -> (double precision float=w50:dbl)
      n3 = To Double Precision Float(number=w32) -> (double precision float=w34:dbl)
      n4 = To Double Precision Float(number=w16) -> (double precision float=w18:dbl)
      n5 = Divide(x="Sampling freuqncy(Hz)", y=w50) -> (x/y=w38:dbl)
      n6 = Format Into String(format string="%04b" ("포맷 문자열"), "User number") -> (resulting string=w27:string)  [unwired: 2 in, 1 out]
      n7 = Reciprocal(x=w34) -> (1/x=w33:dbl)
      n8 = Reciprocal(x=w18) -> (1/x=w17:dbl)
      n9 = call "CodeConvert(SubVI).vi"("Code"=w27) -> ("Code_array"=w25:dbl[])
      n10 = Divide(x=30000.0, y="Sampling freuqncy(Hz)") -> (x/y=w42:dbl)
      n11 = Initialize Array(w33, w32) -> (w31:dbl[])
      n12 = call "ChirpSourceGen(SubVI).vi"("Frequency2(Hz)"="Stop frequency(Hz)", "Frequency1(Hz)"="Start frequency(Hz)", "Pulse length(sec)"="Symbol length(sec)", "Fs(Hz)"=w38) -> ("M.F. Tap(F2-1)"=w35:dbl[], "M.F. Tap(F1-2)"=w40:dbl[])  [unwired: 1 out]
      n13 = call "ChirpSourceGen(SubVI).vi"("Frequency2(Hz)"="Stop frequency(Hz) 2", "Frequency1(Hz)"="Start frequency(Hz) 2", "Pulse length(sec)"="Symbol length(sec)", "Fs(Hz)"="Sampling freuqncy(Hz) 2") -> ("M.F. Tap(F2-1)"=→"Coefficient2_bit1":dbl[], "M.F. Tap(F1-2)"=→"Coefficient2_bit0":dbl[])  [unwired: 1 out]
      n14 = Initialize Array(w17, w16) -> (→"MovingAverage_Coefficient":dbl[])
      n15 = Insert Into Array(array=dbl[] [0.0, 1.0], new element #1=w25, new element #2=dbl[] [1.0, 0.0]) -> (w23:dbl[])  [unwired: 1 in]
      "Target code" <- w23
      n16 = call <vilib>:"Sine Wave.vi"("samples"="Number of sample", "amplitude"=5.0, "frequency"=w42) -> ("sine wave"=w39:dbl[])  [unwired: 2 in, 2 out]
    }
    frame #1 {
      n17 = while {
        tunnel: w62 -> [w75]
        tunnel: w61 -> [w74]
        tunnel: w60 -> [w73]
        tunnel: w59 -> [w72]
        tunnel: w58 -> [w71]
        tunnel: w57 -> [w70]
        tunnel: w56 -> [w69]
        tunnel: w55 -> [w68]
        tunnel: w54 -> [w67]
        tunnel: w53 -> [w66]
        tunnel: w52 -> [w65]
        tunnel: w51 -> [w64]
        stop <- FALSE stop-if-true
        n18 = flat-sequence {
          tunnel: w71 -> [w105]
          tunnel: [w106] -> w89
          tunnel: w72 -> [w104]
          tunnel: [w104] -> w88
          tunnel: w73 -> [w102]
          tunnel: [w102] -> w87
          tunnel: w75 -> [w101]
          tunnel: [w101] -> w86
          tunnel: w74 -> [w103]
          tunnel: [w103] -> w85
          tunnel: [w99] -> w84
          tunnel: [w100] -> w83
          tunnel: w70 -> [w100]
          tunnel: w69 -> [w99]
          tunnel: w68 -> [w98]
          tunnel: [w98] -> w82
          tunnel: [w97] -> w81
          tunnel: w67 -> [w97]
          tunnel: [w96] -> w80
          tunnel: w66 -> [w96]
          tunnel: w65 -> [w95]
          tunnel: [w95] -> w79
          tunnel: [w94] -> w78
          tunnel: w64 -> [w94]
          tunnel: w89 -> [w150]
          tunnel: w88 -> [w149]
          tunnel: w87 -> [w148]
          tunnel: w86 -> [w146]
          tunnel: w85 -> [w147]
          tunnel: w84 -> [w135]
          tunnel: w83 -> [w123]
          tunnel: w82 -> [w124]
          tunnel: w81 -> [w108]
          tunnel: w80 -> [w115]
          tunnel: w79 -> [w114]
          tunnel: w78 -> [w109]
          tunnel: [w477] -> w77
          tunnel: [0] -> w76
          tunnel: w77 -> [w480]
          tunnel: w76 -> [w479]
          frame #0 {
            n19 = local write "Signal processing"(FALSE ("Signal processing")) -> ()
            n20 = local write "DoA Estimation"(FALSE ("DoA Estimation")) -> ()
            n21 = call <vilib>:"DAQmx Reset Device.vi"("device in"=w105) -> ("error out"=w106:errorcluster)  [unwired: 1 in, 13 out]
            n22 = local write "Display"(FALSE ("Display")) -> ()
            n23 = local write "Detect"(FALSE ("Detect")) -> ()
          }
          frame #1 {
            w107 = dbl[] [-1.0, -1.0, -1.0, -1.0, -1.0, -1.0, -1.0, -1.0]
            w121 = "Proc1" ("이름(이름없음)")
            w122 = "Proc0" ("이름(이름없음)")
            w120 = dbl[][] []
            w136 = "SIG0" ("이름(이름없음)")
            w143 = waveform(dbl) {"t0"=timestamp(0 s since 1904-01-01), "dt"=1.0, "Y"=[]} ("Waveform")
            w126 = "SIG1" ("이름(이름없음)")
            # "buffer"
            # "Target code"
            # "[Post processing]  1. Queue get : Proc0, Proc1 / 2. Threshold estimation with moving average / 3. Peak and valley detection / 4. Demodulation"
            # "[Signal processing]\n1. Queue get : SIG1\n2. Data type converting : Waveform (DBL) --> Array (DBL)\n3. DDC (Digital to Digital Convering)\n  - DSB modulation : Multiply carrier signal (30kHz)\n  - Decimate : 192kHz sample rate --> 16kHz sample rate\n4. Cross-correlation with down-chirp (4k ~ 0Hz)\n5. Envelope detection (Hilbert transform) & square\n6. Queue put : Proc1"
            # "[Signal processing]\n1. Queue get : SIG0\n2. Data type converting : Waveform (DBL) --> Array (DBL)\n3. DDC (Digital to Digital Convering)\n  - DSB modulation : Multiply carrier signal (30kHz)\n  - Decimate : 192kHz sample rate --> 16kHz sample rate\n4. Cross-correlation with up-chirp (0 ~ 4kHz)\n5. Envelope detection (Hilbert transform) & square\n6. Queue put : Proc0"
            # "[Data Acquistion (ADC)]\n1. Device reset\n2. Creat channel\n3, Set sample clock\n  - Sampling frequency : 192kHz\n  - Number of sample (Chunk size) : 38400\n4. Start task\n5. Data read\n6. Queue put : SIG0, SIG1\n  - Queue data type : Waveform (DBL)"
            # "Moving average prameter based on FIR filter calculation"
            # "Coefficient for bit 1 : Down-chirp"
            # "Coefficient for bit 0 : Up-chirp"
            # "Decimation rate"
            # "Carrier signal"
            n24 = call-poly <vilib>:"DAQmx Create Virtual Channel.vi"("physical channels"=w149, "error in"=w150) -> ("task out"=w152:refnum<k21>, "error out"=w151:errorcluster)  [unwired: 7 in, 5 out]
            n25 = call-poly <vilib>:"DAQmx Timing.vi"("task/channels in"=w152, "sample mode"=w147, "samples per channel"=w146, "rate"=w148, "error in"=w151) -> ("task out"=w153:refnum<k21>, "error out"=w154:errorcluster)  [unwired: 2 in, 7 out]
            n26 = call <vilib>:"DAQmx Start Task.vi"("task/channels in"=w153, "error in"=w154) -> ("task out"=w155:refnum<k21>, "error out"=w156:errorcluster)  [unwired: 12 in]
            n27 = Build Array(w143, w143, w143, w143, w143, w143, w143, w143) -> (w125:waveform(dbl)[])
            n28 = Obtain Queue(name (unnamed)=w126, element data type=w125) -> (queue out=w145:refnum<queue>, error out=w144:errorcluster)  [unwired: 3 in, 1 out]
            n29 = Obtain Queue(name (unnamed)=w136, element data type=w125) -> (queue out=w142:refnum<queue>, error out=w141:errorcluster)  [unwired: 3 in, 1 out]
            n30 = while {
              tunnel: w155 -> [w452]
              tunnel: w156 -> [w451]
              tunnel: [w450] -> w159
              tunnel: [w449] -> w160
              tunnel: w146 -> [w448]
              tunnel: w145 -> [w447]
              tunnel: w144 -> [w446]
              tunnel: w142 -> [w445]
              tunnel: w141 -> [w444]
              stop <- w442 stop-if-true
              # "Queue\nput"
              n31 = call-poly <vilib>:"DAQmx Read.vi"("task/channels in"=w452, "number of samples per channel"=w448, "error in"=w451) -> ("task out"=w450:refnum<k21>, "data"=w443:waveform(dbl)[], "error out"=w449:errorcluster)  [unwired: 10 out]
              n32 = Enqueue Element(queue=w445, element=w443, error in (no error)=w444) -> ()  [unwired: 1 in, 3 out]
              n33 = Enqueue Element(queue=w447, element=w443, error in (no error)=w446) -> ()  [unwired: 1 in, 3 out]
              n34 = local read "Detect"() -> (w442:bool)
            }
            n35 = call <vilib>:"DAQmx Stop Task.vi"("task/channels in"=w159, "error in"=w160) -> ("task out"=w158:refnum<k21>, "error out"=w157:errorcluster)  [unwired: 12 out]
            n36 = call <vilib>:"DAQmx Clear Task.vi"("task in"=w158, "error in"=w157) -> ()  [unwired: 14 out]
            n37 = Obtain Queue(name (unnamed)=w122, element data type=w120) -> (queue out=w140:refnum<queue>, error out=w139:errorcluster)  [unwired: 3 in, 1 out]
            n38 = Obtain Queue(name (unnamed)=w136, element data type=w125) -> (queue out=w138:refnum<queue>, error out=w137:errorcluster)  [unwired: 3 in, 1 out]
            n39 = while {
              tunnel: w138 -> [w441]
              tunnel: w137 -> [w440]
              tunnel: w140 -> [w439]
              tunnel: w139 -> [w438]
              tunnel: [w437] -> w134
              tunnel: [w436] -> w133
              tunnel: w124 -> [w376]
              tunnel: w123 -> [w375]
              tunnel: w135 -> [w374]
              stop <- w372 stop-if-true
              w386 = TRUE ("averaging")
              w435 = TRUE ("init/cont (init:F)")
              # "Queue\nput"
              # "Queue\nget"
              # "Envelope\nwith hilbert"
              # "Cross\ncorrelation"
              # "Decimate"
              # "DDC"
              n40 = Dequeue Element(queue=w441, error in (no error)=w440) -> (queue out=w437:refnum<queue>, element=w377:waveform(dbl)[], error out=w436:errorcluster)  [unwired: 2 out]
              n41 = Index Array(array=w377) -> (element #1=w434:waveform(dbl), element #2=w433:waveform(dbl), element #3=w432:waveform(dbl), element #4=w431:waveform(dbl), element #5=w430:waveform(dbl), element #6=w429:waveform(dbl), element #7=w428:waveform(dbl), element #8=w427:waveform(dbl))  [unwired: 8 in]
              n42 = Unbundle By Name(w434) -> ("Y"=w426:dbl[])
              n43 = Unbundle By Name(w433) -> ("Y"=w425:dbl[])
              n44 = Unbundle By Name(w432) -> ("Y"=w424:dbl[])
              n45 = Unbundle By Name(w431) -> ("Y"=w423:dbl[])
              n46 = Unbundle By Name(w430) -> ("Y"=w422:dbl[])
              n47 = Unbundle By Name(w429) -> ("Y"=w421:dbl[])
              n48 = Unbundle By Name(w428) -> ("Y"=w420:dbl[])
              n49 = Unbundle By Name(w427) -> ("Y"=w419:dbl[])
              n50 = Multiply(x=w426, y=w376) -> (x*y=w401:dbl[])
              n51 = Multiply(x=w425, y=w376) -> (x*y=w400:dbl[])
              n52 = Multiply(x=w424, y=w376) -> (x*y=w399:dbl[])
              n53 = Multiply(x=w423, y=w376) -> (x*y=w398:dbl[])
              n54 = Multiply(x=w422, y=w376) -> (x*y=w397:dbl[])
              n55 = Multiply(x=w421, y=w376) -> (x*y=w396:dbl[])
              n56 = Multiply(x=w420, y=w376) -> (x*y=w395:dbl[])
              n57 = Multiply(x=w419, y=w376) -> (x*y=w394:dbl[])
              n58 = call-poly <vilib>:"Decimate (single shot).vi"("averaging"=w386, "decimating factor"=w375, "X"=w396) -> ("Decimated Array"=w389:dbl[])  [unwired: 7 in, 1 out]
              n59 = call-poly <vilib>:"Decimate (single shot).vi"("averaging"=w386, "decimating factor"=w375, "X"=w394) -> ("Decimated Array"=w387:dbl[])  [unwired: 7 in, 1 out]
              n60 = call-poly <vilib>:"Decimate (single shot).vi"("averaging"=w386, "decimating factor"=w375, "X"=w400) -> ("Decimated Array"=w393:dbl[])  [unwired: 7 in, 1 out]
              n61 = call-poly <vilib>:"Decimate (single shot).vi"("averaging"=w386, "decimating factor"=w375, "X"=w398) -> ("Decimated Array"=w391:dbl[])  [unwired: 7 in, 1 out]
              n62 = call-poly <vilib>:"Decimate (single shot).vi"("averaging"=w386, "decimating factor"=w375, "X"=w397) -> ("Decimated Array"=w390:dbl[])  [unwired: 7 in, 1 out]
              n63 = call-poly <vilib>:"Decimate (single shot).vi"("averaging"=w386, "decimating factor"=w375, "X"=w395) -> ("Decimated Array"=w388:dbl[])  [unwired: 7 in, 1 out]
              n64 = call-poly <vilib>:"Decimate (single shot).vi"("averaging"=w386, "decimating factor"=w375, "X"=w401) -> ("Decimated Array"=w402:dbl[])  [unwired: 7 in, 1 out]
              n65 = call-poly <vilib>:"Decimate (single shot).vi"("averaging"=w386, "decimating factor"=w375, "X"=w399) -> ("Decimated Array"=w392:dbl[])  [unwired: 7 in, 1 out]
              n66 = call-poly <vilib>:"FIR Filter.vi"("init/cont (init:F)"=w435, "FIR Coefficients"=w374, "X"=w402) -> ("Filtered X"=w418:dbl[])  [unwired: 1 in, 1 out]
              n67 = call-poly <vilib>:"FIR Filter.vi"("init/cont (init:F)"=w435, "FIR Coefficients"=w374, "X"=w393) -> ("Filtered X"=w417:dbl[])  [unwired: 1 in, 1 out]
              n68 = call-poly <vilib>:"FIR Filter.vi"("init/cont (init:F)"=w435, "FIR Coefficients"=w374, "X"=w392) -> ("Filtered X"=w416:dbl[])  [unwired: 1 in, 1 out]
              n69 = call-poly <vilib>:"FIR Filter.vi"("init/cont (init:F)"=w435, "FIR Coefficients"=w374, "X"=w391) -> ("Filtered X"=w415:dbl[])  [unwired: 1 in, 1 out]
              n70 = call-poly <vilib>:"FIR Filter.vi"("init/cont (init:F)"=w435, "FIR Coefficients"=w374, "X"=w390) -> ("Filtered X"=w414:dbl[])  [unwired: 1 in, 1 out]
              n71 = call-poly <vilib>:"FIR Filter.vi"("init/cont (init:F)"=w435, "FIR Coefficients"=w374, "X"=w389) -> ("Filtered X"=w413:dbl[])  [unwired: 1 in, 1 out]
              n72 = call-poly <vilib>:"FIR Filter.vi"("init/cont (init:F)"=w435, "FIR Coefficients"=w374, "X"=w388) -> ("Filtered X"=w412:dbl[])  [unwired: 1 in, 1 out]
              n73 = call-poly <vilib>:"FIR Filter.vi"("init/cont (init:F)"=w435, "FIR Coefficients"=w374, "X"=w387) -> ("Filtered X"=w411:dbl[])  [unwired: 1 in, 1 out]
              n74 = call "Envelope(SubVI).vi"("x"=w418) -> ("Y"=w410:dbl[])
              n75 = call "Envelope(SubVI).vi"("x"=w417) -> ("Y"=w409:dbl[])
              n76 = call "Envelope(SubVI).vi"("x"=w416) -> ("Y"=w408:dbl[])
              n77 = call "Envelope(SubVI).vi"("x"=w415) -> ("Y"=w407:dbl[])
              n78 = call "Envelope(SubVI).vi"("x"=w414) -> ("Y"=w406:dbl[])
              n79 = call "Envelope(SubVI).vi"("x"=w413) -> ("Y"=w405:dbl[])
              n80 = call "Envelope(SubVI).vi"("x"=w412) -> ("Y"=w404:dbl[])
              n81 = call "Envelope(SubVI).vi"("x"=w411) -> ("Y"=w403:dbl[])
              n82 = Square(x=w410) -> (x^2=w385:dbl[])
              n83 = Square(x=w409) -> (x^2=w384:dbl[])
              n84 = Square(x=w408) -> (x^2=w383:dbl[])
              n85 = Square(x=w407) -> (x^2=w382:dbl[])
              n86 = Square(x=w406) -> (x^2=w381:dbl[])
              n87 = Square(x=w405) -> (x^2=w380:dbl[])
              n88 = Square(x=w404) -> (x^2=w379:dbl[])
              n89 = Square(x=w403) -> (x^2=w378:dbl[])
              n90 = local read "Detect"() -> (w372:bool)
              n91 = Build Array(w385, w384, w383, w382, w381, w380, w379, w378) -> (w373:dbl[][])
              n92 = Enqueue Element(queue=w439, element=w373, error in (no error)=w438) -> ()  [unwired: 1 in, 3 out]
            }
            n93 = Release Queue(queue=w134, error in (no error)=w133) -> ()  [unwired: 1 in, 3 out]
            n94 = Obtain Queue(name (unnamed)=w121, element data type=w120) -> (queue out=w132:refnum<queue>, error out=w131:errorcluster)  [unwired: 3 in, 1 out]
            n95 = Obtain Queue(name (unnamed)=w126, element data type=w125) -> (queue out=w130:refnum<queue>, error out=w129:errorcluster)  [unwired: 3 in, 1 out]
            n96 = while {
              tunnel: w130 -> [w371]
              tunnel: w129 -> [w370]
              tunnel: w132 -> [w369]
              tunnel: w131 -> [w368]
              tunnel: [w367] -> w128
              tunnel: [w366] -> w127
              tunnel: w124 -> [w306]
              tunnel: w123 -> [w305]
              tunnel: w108 -> [w304]
              stop <- w302 stop-if-true
              w316 = TRUE ("averaging")
              w365 = TRUE ("init/cont (init:F)")
              # "Queue\nput"
              # "Queue\nget"
              # "Envelope\nwith hilbert"
              # "Cross\ncorrelation"
              # "Decimate"
              # "DDC"
              n97 = Dequeue Element(queue=w371, error in (no error)=w370) -> (queue out=w367:refnum<queue>, element=w307:waveform(dbl)[], error out=w366:errorcluster)  [unwired: 2 out]
              n98 = Index Array(array=w307) -> (element #1=w364:waveform(dbl), element #2=w363:waveform(dbl), element #3=w362:waveform(dbl), element #4=w361:waveform(dbl), element #5=w360:waveform(dbl), element #6=w359:waveform(dbl), element #7=w358:waveform(dbl), element #8=w357:waveform(dbl))  [unwired: 8 in]
              n99 = Unbundle By Name(w364) -> ("Y"=w356:dbl[])
              n100 = Unbundle By Name(w363) -> ("Y"=w355:dbl[])
              n101 = Unbundle By Name(w362) -> ("Y"=w354:dbl[])
              n102 = Unbundle By Name(w361) -> ("Y"=w353:dbl[])
              n103 = Unbundle By Name(w360) -> ("Y"=w352:dbl[])
              n104 = Unbundle By Name(w359) -> ("Y"=w351:dbl[])
              n105 = Unbundle By Name(w358) -> ("Y"=w350:dbl[])
              n106 = Unbundle By Name(w357) -> ("Y"=w349:dbl[])
              n107 = Multiply(x=w356, y=w306) -> (x*y=w331:dbl[])
              n108 = Multiply(x=w355, y=w306) -> (x*y=w330:dbl[])
              n109 = Multiply(x=w354, y=w306) -> (x*y=w329:dbl[])
              n110 = Multiply(x=w353, y=w306) -> (x*y=w328:dbl[])
              n111 = Multiply(x=w352, y=w306) -> (x*y=w327:dbl[])
              n112 = Multiply(x=w351, y=w306) -> (x*y=w326:dbl[])
              n113 = Multiply(x=w350, y=w306) -> (x*y=w325:dbl[])
              n114 = Multiply(x=w349, y=w306) -> (x*y=w324:dbl[])
              n115 = call-poly <vilib>:"Decimate (single shot).vi"("averaging"=w316, "decimating factor"=w305, "X"=w326) -> ("Decimated Array"=w319:dbl[])  [unwired: 7 in, 1 out]
              n116 = call-poly <vilib>:"Decimate (single shot).vi"("averaging"=w316, "decimating factor"=w305, "X"=w324) -> ("Decimated Array"=w317:dbl[])  [unwired: 7 in, 1 out]
              n117 = call-poly <vilib>:"Decimate (single shot).vi"("averaging"=w316, "decimating factor"=w305, "X"=w330) -> ("Decimated Array"=w323:dbl[])  [unwired: 7 in, 1 out]
              n118 = call-poly <vilib>:"Decimate (single shot).vi"("averaging"=w316, "decimating factor"=w305, "X"=w328) -> ("Decimated Array"=w321:dbl[])  [unwired: 7 in, 1 out]
              n119 = call-poly <vilib>:"Decimate (single shot).vi"("averaging"=w316, "decimating factor"=w305, "X"=w327) -> ("Decimated Array"=w320:dbl[])  [unwired: 7 in, 1 out]
              n120 = call-poly <vilib>:"Decimate (single shot).vi"("averaging"=w316, "decimating factor"=w305, "X"=w325) -> ("Decimated Array"=w318:dbl[])  [unwired: 7 in, 1 out]
              n121 = call-poly <vilib>:"Decimate (single shot).vi"("averaging"=w316, "decimating factor"=w305, "X"=w331) -> ("Decimated Array"=w332:dbl[])  [unwired: 7 in, 1 out]
              n122 = call-poly <vilib>:"Decimate (single shot).vi"("averaging"=w316, "decimating factor"=w305, "X"=w329) -> ("Decimated Array"=w322:dbl[])  [unwired: 7 in, 1 out]
              n123 = call-poly <vilib>:"FIR Filter.vi"("init/cont (init:F)"=w365, "FIR Coefficients"=w304, "X"=w332) -> ("Filtered X"=w348:dbl[])  [unwired: 1 in, 1 out]
              n124 = call-poly <vilib>:"FIR Filter.vi"("init/cont (init:F)"=w365, "FIR Coefficients"=w304, "X"=w323) -> ("Filtered X"=w347:dbl[])  [unwired: 1 in, 1 out]
              n125 = call-poly <vilib>:"FIR Filter.vi"("init/cont (init:F)"=w365, "FIR Coefficients"=w304, "X"=w322) -> ("Filtered X"=w346:dbl[])  [unwired: 1 in, 1 out]
              n126 = call-poly <vilib>:"FIR Filter.vi"("init/cont (init:F)"=w365, "FIR Coefficients"=w304, "X"=w321) -> ("Filtered X"=w345:dbl[])  [unwired: 1 in, 1 out]
              n127 = call-poly <vilib>:"FIR Filter.vi"("init/cont (init:F)"=w365, "FIR Coefficients"=w304, "X"=w320) -> ("Filtered X"=w344:dbl[])  [unwired: 1 in, 1 out]
              n128 = call-poly <vilib>:"FIR Filter.vi"("init/cont (init:F)"=w365, "FIR Coefficients"=w304, "X"=w319) -> ("Filtered X"=w343:dbl[])  [unwired: 1 in, 1 out]
              n129 = call-poly <vilib>:"FIR Filter.vi"("init/cont (init:F)"=w365, "FIR Coefficients"=w304, "X"=w318) -> ("Filtered X"=w342:dbl[])  [unwired: 1 in, 1 out]
              n130 = call-poly <vilib>:"FIR Filter.vi"("init/cont (init:F)"=w365, "FIR Coefficients"=w304, "X"=w317) -> ("Filtered X"=w341:dbl[])  [unwired: 1 in, 1 out]
              n131 = call "Envelope(SubVI).vi"("x"=w348) -> ("Y"=w340:dbl[])
              n132 = call "Envelope(SubVI).vi"("x"=w347) -> ("Y"=w339:dbl[])
              n133 = call "Envelope(SubVI).vi"("x"=w346) -> ("Y"=w338:dbl[])
              n134 = call "Envelope(SubVI).vi"("x"=w345) -> ("Y"=w337:dbl[])
              n135 = call "Envelope(SubVI).vi"("x"=w344) -> ("Y"=w336:dbl[])
              n136 = call "Envelope(SubVI).vi"("x"=w343) -> ("Y"=w335:dbl[])
              n137 = call "Envelope(SubVI).vi"("x"=w342) -> ("Y"=w334:dbl[])
              n138 = call "Envelope(SubVI).vi"("x"=w341) -> ("Y"=w333:dbl[])
              n139 = Square(x=w340) -> (x^2=w315:dbl[])
              n140 = Square(x=w339) -> (x^2=w314:dbl[])
              n141 = Square(x=w338) -> (x^2=w313:dbl[])
              n142 = Square(x=w337) -> (x^2=w312:dbl[])
              n143 = Square(x=w336) -> (x^2=w311:dbl[])
              n144 = Square(x=w335) -> (x^2=w310:dbl[])
              n145 = Square(x=w334) -> (x^2=w309:dbl[])
              n146 = Square(x=w333) -> (x^2=w308:dbl[])
              n147 = local read "Detect"() -> (w302:bool)
              n148 = Build Array(w315, w314, w313, w312, w311, w310, w309, w308) -> (w303:dbl[][])
              n149 = Enqueue Element(queue=w369, element=w303, error in (no error)=w368) -> ()  [unwired: 1 in, 3 out]
            }
            n150 = Release Queue(queue=w128, error in (no error)=w127) -> ()  [unwired: 1 in, 3 out]
            n151 = Obtain Queue(name (unnamed)=w122, element data type=w120) -> (queue out=w119:refnum<queue>, error out=w118:errorcluster)  [unwired: 3 in, 1 out]
            n152 = Obtain Queue(name (unnamed)=w121, element data type=w120) -> (queue out=w117:refnum<queue>, error out=w116:errorcluster)  [unwired: 3 in, 1 out]
            n153 = while {
              tunnel: w119 -> [w301]
              tunnel: w118 -> [w300]
              tunnel: w117 -> [w299]
              tunnel: w116 -> [w298]
              tunnel: w115 -> [w296]
              tunnel: w114 -> [w260]
              tunnel: [w208] -> w113
              tunnel: [w207] -> w112
              tunnel: [w206] -> w111
              tunnel: [w205] -> w110
              tunnel: w109 -> [w204]
              shift-right: [w168] -> _
              shift-left: w107 -> [w184]
              shift-right: [w167] -> _
              shift-left: w107 -> [w183]
              shift-right: [w166] -> _
              shift-left: w107 -> [w182]
              shift-right: [w165] -> _
              shift-left: w107 -> [w181]
              shift-right: [w164] -> _
              shift-left: w107 -> [w180]
              shift-right: [w163] -> _
              shift-left: w107 -> [w179]
              shift-right: [w162] -> _
              shift-left: w107 -> [w178]
              shift-right: [w161] -> _
              shift-left: w107 -> [w177]
              stop <- w193 stop-if-true
              w285 = enum32{"Peaks", "Valleys"}."Valleys" ("peaks/valleys")
              w286 = enum32{"Peaks", "Valleys"}."Peaks" ("peaks/valleys")
              w284 = 5 ("width")
              w295 = TRUE ("init/cont (init:F)")
              # "If code detected, Break!"
              # "Decision"
              # "Peak / Valley detection"
              # "Queue\nget"
              # "Threshold\nestimation"
              # "Moving\naverage"
              n154 = Dequeue Element(queue=w301, error in (no error)=w300) -> (queue out=w208:refnum<queue>, element=w242:dbl[][], error out=w207:errorcluster)  [unwired: 2 out]
              n155 = Dequeue Element(queue=w299, error in (no error)=w298) -> (queue out=w206:refnum<queue>, element=w241:dbl[][], error out=w205:errorcluster)  [unwired: 2 out]
              n156 = Subtract(x=w242, y=w241) -> (x-y=w297:dbl[][])
              n157 = Index Array(array=w297) -> (element #1=w283:dbl[], element #2=w282:dbl[], element #3=w281:dbl[], element #4=w280:dbl[], element #5=w279:dbl[], element #6=w278:dbl[], element #7=w277:dbl[], element #8=w245:dbl[])  [unwired: 16 in]
              n158 = call-poly <vilib>:"FIR Filter.vi"("init/cont (init:F)"=w295, "FIR Coefficients"=w296, "X"=w283) -> ("Filtered X"=w294:dbl[])  [unwired: 1 in, 1 out]
              n159 = call-poly <vilib>:"FIR Filter.vi"("init/cont (init:F)"=w295, "FIR Coefficients"=w296, "X"=w282) -> ("Filtered X"=w293:dbl[])  [unwired: 1 in, 1 out]
              n160 = call-poly <vilib>:"FIR Filter.vi"("init/cont (init:F)"=w295, "FIR Coefficients"=w296, "X"=w281) -> ("Filtered X"=w292:dbl[])  [unwired: 1 in, 1 out]
              n161 = call-poly <vilib>:"FIR Filter.vi"("init/cont (init:F)"=w295, "FIR Coefficients"=w296, "X"=w280) -> ("Filtered X"=w291:dbl[])  [unwired: 1 in, 1 out]
              n162 = call-poly <vilib>:"FIR Filter.vi"("init/cont (init:F)"=w295, "FIR Coefficients"=w296, "X"=w279) -> ("Filtered X"=w290:dbl[])  [unwired: 1 in, 1 out]
              n163 = call-poly <vilib>:"FIR Filter.vi"("init/cont (init:F)"=w295, "FIR Coefficients"=w296, "X"=w278) -> ("Filtered X"=w289:dbl[])  [unwired: 1 in, 1 out]
              n164 = call-poly <vilib>:"FIR Filter.vi"("init/cont (init:F)"=w295, "FIR Coefficients"=w296, "X"=w277) -> ("Filtered X"=w288:dbl[])  [unwired: 1 in, 1 out]
              n165 = call-poly <vilib>:"FIR Filter.vi"("init/cont (init:F)"=w295, "FIR Coefficients"=w296, "X"=w245) -> ("Filtered X"=w287:dbl[])  [unwired: 1 in, 1 out]
              n166 = Array Max & Min(array=w294) -> (max value=w276:dbl, min value=w275:dbl)  [unwired: 2 out]
              n167 = Array Max & Min(array=w293) -> (max value=w274:dbl, min value=w273:dbl)  [unwired: 2 out]
              n168 = Array Max & Min(array=w292) -> (max value=w272:dbl, min value=w271:dbl)  [unwired: 2 out]
              n169 = Array Max & Min(array=w291) -> (max value=w270:dbl, min value=w269:dbl)  [unwired: 2 out]
              n170 = Array Max & Min(array=w290) -> (max value=w268:dbl, min value=w267:dbl)  [unwired: 2 out]
              n171 = Array Max & Min(array=w289) -> (max value=w266:dbl, min value=w265:dbl)  [unwired: 2 out]
              n172 = Array Max & Min(array=w288) -> (max value=w264:dbl, min value=w263:dbl)  [unwired: 2 out]
              n173 = Array Max & Min(array=w287) -> (max value=w262:dbl, min value=w261:dbl)  [unwired: 2 out]
              n174 = call "ThresholdEstimation(SubVI).vi"("Margin"=w260, "최소값"=w273, "최대값"=w274) -> ("N.Th"=w247:dbl, "P.Th"=w258:dbl)
              n175 = call "ThresholdEstimation(SubVI).vi"("Margin"=w260, "최소값"=w271, "최대값"=w272) -> ("N.Th"=w248:dbl, "P.Th"=w257:dbl)
              n176 = call "ThresholdEstimation(SubVI).vi"("Margin"=w260, "최소값"=w269, "최대값"=w270) -> ("N.Th"=w249:dbl, "P.Th"=w256:dbl)
              n177 = call "ThresholdEstimation(SubVI).vi"("Margin"=w260, "최소값"=w267, "최대값"=w268) -> ("N.Th"=w250:dbl, "P.Th"=w255:dbl)
              n178 = call "ThresholdEstimation(SubVI).vi"("Margin"=w260, "최소값"=w275, "최대값"=w276) -> ("N.Th"=w246:dbl, "P.Th"=w259:dbl)
              n179 = call "ThresholdEstimation(SubVI).vi"("Margin"=w260, "최소값"=w265, "최대값"=w266) -> ("N.Th"=w251:dbl, "P.Th"=w254:dbl)
              n180 = call "ThresholdEstimation(SubVI).vi"("Margin"=w260, "최소값"=w263, "최대값"=w264) -> ("N.Th"=w252:dbl, "P.Th"=w253:dbl)
              n181 = call "ThresholdEstimation(SubVI).vi"("Margin"=w260, "최소값"=w261, "최대값"=w262) -> ("N.Th"=w244:dbl, "P.Th"=w243:dbl)
              n182 = call <vilib>:"Peak Detector.vi"("peaks/valleys"=w286, "width"=w284, "threshold"=w259, "X"=w283) -> ("Locations"=w217:dbl[], "# found"=w233:i32)  [unwired: 3 in, 3 out]
              n183 = call <vilib>:"Peak Detector.vi"("peaks/valleys"=w286, "width"=w284, "threshold"=w258, "X"=w282) -> ("Locations"=w218:dbl[], "# found"=w234:i32)  [unwired: 3 in, 3 out]
              n184 = call <vilib>:"Peak Detector.vi"("peaks/valleys"=w286, "width"=w284, "threshold"=w257, "X"=w281) -> ("Locations"=w219:dbl[], "# found"=w235:i32)  [unwired: 3 in, 3 out]
              n185 = call <vilib>:"Peak Detector.vi"("peaks/valleys"=w286, "width"=w284, "threshold"=w256, "X"=w280) -> ("Locations"=w220:dbl[], "# found"=w236:i32)  [unwired: 3 in, 3 out]
              n186 = call <vilib>:"Peak Detector.vi"("peaks/valleys"=w286, "width"=w284, "threshold"=w255, "X"=w279) -> ("Locations"=w221:dbl[], "# found"=w237:i32)  [unwired: 3 in, 3 out]
              n187 = call <vilib>:"Peak Detector.vi"("peaks/valleys"=w286, "width"=w284, "threshold"=w254, "X"=w278) -> ("Locations"=w222:dbl[], "# found"=w238:i32)  [unwired: 3 in, 3 out]
              n188 = call <vilib>:"Peak Detector.vi"("peaks/valleys"=w286, "width"=w284, "threshold"=w253, "X"=w277) -> ("Locations"=w223:dbl[], "# found"=w239:i32)  [unwired: 3 in, 3 out]
              n189 = call <vilib>:"Peak Detector.vi"("peaks/valleys"=w286, "width"=w284, "threshold"=w243, "X"=w245) -> ("Locations"=w224:dbl[], "# found"=w240:i32)  [unwired: 3 in, 3 out]
              n190 = call <vilib>:"Peak Detector.vi"("peaks/valleys"=w285, "width"=w284, "threshold"=w246, "X"=w283) -> ("Locations"=w216:dbl[], "# found"=w232:i32)  [unwired: 3 in, 3 out]
              n191 = call <vilib>:"Peak Detector.vi"("peaks/valleys"=w285, "width"=w284, "threshold"=w247, "X"=w282) -> ("Locations"=w215:dbl[], "# found"=w231:i32)  [unwired: 3 in, 3 out]
              n192 = call <vilib>:"Peak Detector.vi"("peaks/valleys"=w285, "width"=w284, "threshold"=w248, "X"=w281) -> ("Locations"=w214:dbl[], "# found"=w230:i32)  [unwired: 3 in, 3 out]
              n193 = call <vilib>:"Peak Detector.vi"("peaks/valleys"=w285, "width"=w284, "threshold"=w249, "X"=w280) -> ("Locations"=w213:dbl[], "# found"=w229:i32)  [unwired: 3 in, 3 out]
              n194 = call <vilib>:"Peak Detector.vi"("peaks/valleys"=w285, "width"=w284, "threshold"=w250, "X"=w279) -> ("Locations"=w212:dbl[], "# found"=w228:i32)  [unwired: 3 in, 3 out]
              n195 = call <vilib>:"Peak Detector.vi"("peaks/valleys"=w285, "width"=w284, "threshold"=w251, "X"=w278) -> ("Locations"=w211:dbl[], "# found"=w227:i32)  [unwired: 3 in, 3 out]
              n196 = call <vilib>:"Peak Detector.vi"("peaks/valleys"=w285, "width"=w284, "threshold"=w252, "X"=w277) -> ("Locations"=w210:dbl[], "# found"=w226:i32)  [unwired: 3 in, 3 out]
              n197 = call <vilib>:"Peak Detector.vi"("peaks/valleys"=w285, "width"=w284, "threshold"=w244, "X"=w245) -> ("Locations"=w209:dbl[], "# found"=w225:i32)  [unwired: 3 in, 3 out]
              n198 = call "Decision(SubVI).vi"("L_ind0"=w233, "L_ind1"=w232, "Peak_ind0"=w217, "Peak_ind1"=w216) -> ("L_sum"=w176:i32, "Bits"=w192:dbl[])  [unwired: 2 in]
              n199 = call "Decision(SubVI).vi"("L_ind0"=w234, "L_ind1"=w231, "Peak_ind0"=w218, "Peak_ind1"=w215) -> ("L_sum"=w175:i32, "Bits"=w191:dbl[])  [unwired: 2 in]
              n200 = call "Decision(SubVI).vi"("L_ind0"=w235, "L_ind1"=w230, "Peak_ind0"=w219, "Peak_ind1"=w214) -> ("L_sum"=w174:i32, "Bits"=w190:dbl[])  [unwired: 2 in]
              n201 = call "Decision(SubVI).vi"("L_ind0"=w236, "L_ind1"=w229, "Peak_ind0"=w220, "Peak_ind1"=w213) -> ("L_sum"=w173:i32, "Bits"=w189:dbl[])  [unwired: 2 in]
              n202 = call "Decision(SubVI).vi"("L_ind0"=w237, "L_ind1"=w228, "Peak_ind0"=w221, "Peak_ind1"=w212) -> ("L_sum"=w172:i32, "Bits"=w188:dbl[])  [unwired: 2 in]
              n203 = call "Decision(SubVI).vi"("L_ind0"=w238, "L_ind1"=w227, "Peak_ind0"=w222, "Peak_ind1"=w211) -> ("L_sum"=w171:i32, "Bits"=w187:dbl[])  [unwired: 2 in]
              n204 = call "Decision(SubVI).vi"("L_ind0"=w239, "L_ind1"=w226, "Peak_ind0"=w223, "Peak_ind1"=w210) -> ("L_sum"=w170:i32, "Bits"=w186:dbl[])  [unwired: 2 in]
              n205 = call "Decision(SubVI).vi"("L_ind0"=w240, "L_ind1"=w225, "Peak_ind0"=w224, "Peak_ind1"=w209) -> ("L_sum"=w169:i32, "Bits"=w185:dbl[])  [unwired: 2 in]
              n206 = call "DataBuffer(SubVI).vi"("Bits"=w192, "Buffer"=w184) -> ("Data"=w168:dbl[])  [unwired: 2 in]
              n207 = call "DataBuffer(SubVI).vi"("Bits"=w191, "Buffer"=w183) -> ("Data"=w167:dbl[])  [unwired: 2 in]
              n208 = call "DataBuffer(SubVI).vi"("Bits"=w190, "Buffer"=w182) -> ("Data"=w166:dbl[])  [unwired: 2 in]
              n209 = call "DataBuffer(SubVI).vi"("Bits"=w189, "Buffer"=w181) -> ("Data"=w165:dbl[])  [unwired: 2 in]
              n210 = call "DataBuffer(SubVI).vi"("Bits"=w188, "Buffer"=w180) -> ("Data"=w164:dbl[])  [unwired: 2 in]
              n211 = call "DataBuffer(SubVI).vi"("Bits"=w187, "Buffer"=w179) -> ("Data"=w163:dbl[])  [unwired: 2 in]
              n212 = call "DataBuffer(SubVI).vi"("Bits"=w186, "Buffer"=w178) -> ("Data"=w162:dbl[])  [unwired: 2 in]
              n213 = call "DataBuffer(SubVI).vi"("Bits"=w185, "Buffer"=w177) -> ("Data"=w161:dbl[])  [unwired: 2 in]
              n214 = call "CodeDetection(SubVI).vi"("Code"=w204, "Buff"=w168, "L_sum"=w176) -> ("detect"=w203:bool)
              n215 = call "CodeDetection(SubVI).vi"("Code"=w204, "Buff"=w167, "L_sum"=w175) -> ("detect"=w202:bool)
              n216 = call "CodeDetection(SubVI).vi"("Code"=w204, "Buff"=w166, "L_sum"=w174) -> ("detect"=w201:bool)
              n217 = call "CodeDetection(SubVI).vi"("Code"=w204, "Buff"=w165, "L_sum"=w173) -> ("detect"=w200:bool)
              n218 = call "CodeDetection(SubVI).vi"("Code"=w204, "Buff"=w164, "L_sum"=w172) -> ("detect"=w199:bool)
              n219 = call "CodeDetection(SubVI).vi"("Code"=w204, "Buff"=w163, "L_sum"=w171) -> ("detect"=w198:bool)
              n220 = call "CodeDetection(SubVI).vi"("Code"=w204, "Buff"=w162, "L_sum"=w170) -> ("detect"=w197:bool)
              n221 = call "CodeDetection(SubVI).vi"("Code"=w204, "Buff"=w161, "L_sum"=w169) -> ("detect"=w196:bool)
              n222 = Build Array(w203, w202, w201, w200, w199, w198, w197, w196) -> (w195:bool[])
              n223 = Boolean Array To Number(Boolean array=w195) -> (number=w194:u32)
              n224 = Greater Than 0?(x=w194) -> (x > 0?=w193:bool)
              "Detect" <- w193
            }
            n225 = Release Queue(queue=w113, error in (no error)=w112) -> ()  [unwired: 1 in, 3 out]
            n226 = Release Queue(queue=w111, error in (no error)=w110) -> ()  [unwired: 1 in, 3 out]
          }
          frame #2 {
            w454 = dbl[][] []
            w470 = waveform(dbl) {"t0"=timestamp(0 s since 1904-01-01), "dt"=1.0, "Y"=[]} ("Waveform")
            # "Queue clear"
            n227 = local read "Device"() -> (w478:tag)
            n228 = Build Array(w470, w470, w470, w470, w470, w470, w470, w470) -> (w469:waveform(dbl)[])
            n229 = call <vilib>:"DAQmx Reset Device.vi"("device in"=w478) -> ("error out"=w477:errorcluster)  [unwired: 1 in, 13 out]
            n230 = Obtain Queue(name (unnamed)="SIG1" ("이름(이름없음)"), element data type=w469) -> (queue out=w466:refnum<queue>, error out=w465:errorcluster)  [unwired: 3 in, 1 out]
            n231 = Obtain Queue(name (unnamed)="Proc1" ("이름(이름없음)"), element data type=w454) -> (queue out=w458:refnum<queue>, error out=w457:errorcluster)  [unwired: 3 in, 1 out]
            n232 = Obtain Queue(name (unnamed)="SIG0" ("이름(이름없음)"), element data type=w469) -> (queue out=w476:refnum<queue>, error out=w475:errorcluster)  [unwired: 3 in, 1 out]
            n233 = Obtain Queue(name (unnamed)="Proc0" ("이름(이름없음)"), element data type=w454) -> (queue out=w464:refnum<queue>, error out=w463:errorcluster)  [unwired: 3 in, 1 out]
            n234 = Flush Queue(queue=w476, error in (no error)=w475) -> (queue out=w474:refnum<queue>, error out=w473:errorcluster)  [unwired: 1 out]
            n235 = Flush Queue(queue=w466, error in (no error)=w465) -> (queue out=w468:refnum<queue>, error out=w467:errorcluster)  [unwired: 1 out]
            n236 = Flush Queue(queue=w464, error in (no error)=w463) -> (queue out=w462:refnum<queue>, error out=w461:errorcluster)  [unwired: 1 out]
            n237 = Flush Queue(queue=w458, error in (no error)=w457) -> (queue out=w460:refnum<queue>, error out=w459:errorcluster)  [unwired: 1 out]
            n238 = Release Queue(queue=w474, error in (no error)=w473) -> ()  [unwired: 1 in, 3 out]
            n239 = Release Queue(queue=w468, error in (no error)=w467) -> ()  [unwired: 1 in, 3 out]
            n240 = Release Queue(queue=w462, error in (no error)=w461) -> ()  [unwired: 1 in, 3 out]
            n241 = Release Queue(queue=w460, error in (no error)=w459) -> ()  [unwired: 1 in, 3 out]
          }
          frame #3 {
            n242 = while {
              tunnel: w480 -> [w491]
              shift-right: [w488] -> _
              shift-left: w479 -> [w490]
              i -> [w481]
              stop <- w486 stop-if-true
              # "If it is not recognized more than 5 times,"
              n243 = flat-sequence {
                tunnel: w491 -> [w613]
                tunnel: [w517] -> w499
                tunnel: [w516] -> w498
                tunnel: [w515] -> w497
                tunnel: [w514] -> w496
                tunnel: [w513] -> w495
                tunnel: [w512] -> w494
                tunnel: [w511] -> w493
                tunnel: [w510] -> w492
                tunnel: w490 -> [w500]
                tunnel: [w500] -> w489
                tunnel: w499 -> [w1317]
                tunnel: w498 -> [w1316]
                tunnel: w497 -> [w1315]
                tunnel: w496 -> [w1314]
                tunnel: w495 -> [w1313]
                tunnel: w494 -> [w1312]
                tunnel: w493 -> [w1311]
                tunnel: w492 -> [w1310]
                tunnel: w489 -> [w1306]
                tunnel: [w1305] -> w485
                tunnel: [w1304] -> w484
                tunnel: [w1303] -> w483
                tunnel: w485 -> [w1404]
                tunnel: w484 -> [w1448]
                tunnel: w483 -> [w1447]
                tunnel: [w1404] -> w482
                tunnel: [w1494] -> w488
                tunnel: w482 -> [w1494]
                frame #0 {
                  w502 = 1000.0
                  w523 = waveform(dbl) {"t0"=timestamp(0 s since 1904-01-01), "dt"=1.0, "Y"=[]} ("Waveform")
                  w602 = 10123 items=["유한 샘플"=10178, "연속 샘플"=10123, "하드웨어 타이밍에 의한 단일 포인트"=12522] ("sample mode")
                  w606 = 10178 items=["유한 샘플"=10178, "연속 샘플"=10123, "하드웨어 타이밍에 의한 단일 포인트"=12522] ("sample mode")
                  # "Signal porcessing / Code identification"
                  # "Queue\nput"
                  # "[Rx.time]\nTravel time (1km) : 670ms * 2\nDown-link : 210ms\nUp-link : 1024ms\nTotal : Rx.time > 2574ms"
                  # "[Data Acquistion (ADC)]"
                  # "Signal generation (Counter) / delaty time : 200ms"
                  n244 = local read "Sampling freuqncy(Hz) 2"() -> (w555:dbl)
                  n245 = local read "Number of pulse"() -> (w607:i32)
                  n246 = local read "Output terminal"() -> (w610:tag)
                  n247 = local read "Physical channel"() -> (w604:tag)
                  n248 = local read "Frequency(Hz)"() -> (w615:dbl)
                  n249 = local read "Number of sample 2"() -> (w558:i32)
                  n250 = local read "Cycle share"() -> (w614:dbl)
                  n251 = local read "Counter"() -> (w616:tag)
                  n252 = call-poly <vilib>:"DAQmx Create Virtual Channel.vi"("frequency"=w615, "duty cycle"=w614, "counter"=w616, "error in"=w613) -> ("task out"=w612:refnum<k21>, "error out"=w611:errorcluster)  [unwired: 10 in]
                  n253 = call-poly <vilib>:"DAQmx Create Virtual Channel.vi"("physical channels"=w604) -> ("task out"=w603:refnum<k21>, "error out"=w605:errorcluster)  [unwired: 8 in, 5 out]
                  n254 = property class="DAQmx 채널"(reference=w612, error in=w611, "CO.Pulse.Term"=w610) -> (reference out=w609:refnum<k21>, error out=w608:errorcluster)
                  n255 = call-poly <vilib>:"DAQmx Timing.vi"("task/channels in"=w603, "sample mode"=w602, "samples per channel"=w558, "rate"=w555, "error in"=w605) -> ("task out"=w601:refnum<k21>, "error out"=w600:errorcluster)  [unwired: 2 in, 7 out]
                  n256 = call-poly <vilib>:"DAQmx Timing.vi"("task/channels in"=w609, "sample mode"=w606, "samples per channel"=w607, "error in"=w608) -> ("task out"=w599:refnum<k21>, "error out"=w598:errorcluster)  [unwired: 10 in]
                  n257 = flat-sequence {
                    tunnel: w601 -> [w1301]
                    tunnel: w600 -> [w1300]
                    tunnel: w599 -> [w1299]
                    tunnel: w598 -> [w1298]
                    tunnel: [w1299] -> w597
                    tunnel: [w1298] -> w596
                    tunnel: [w1297] -> w588
                    tunnel: [w1296] -> w587
                    frame #0 {
                      n258 = call <vilib>:"DAQmx Start Task.vi"("task/channels in"=w1301, "error in"=w1300) -> ("task out"=w1297:refnum<k21>, "error out"=w1296:errorcluster)  [unwired: 12 in]
                    }
                  }
                  n259 = for {
                    N: 2 -> [_]
                    tunnel: w597 -> [w1294]
                    tunnel: [w1289] -> w594
                    tunnel: w596 -> [w1295]
                    tunnel: [w1288] -> w593
                    # "Delay time"
                    n260 = call <vilib>:"DAQmx Start Task.vi"("task/channels in"=w1294, "error in"=w1295) -> ("task out"=w1293:refnum<k21>, "error out"=w1292:errorcluster)  [unwired: 12 in]
                    n261 = call <vilib>:"DAQmx Is Task Done.vi"("task/channels in"=w1293, "error in"=w1292) -> ("task out"=w1291:refnum<k21>, "error out"=w1290:errorcluster)  [unwired: 11 in, 1 out]
                    n262 = Wait (ms)(milliseconds to wait=u32 200 ("대기 시간 (ms)")) -> ()  [unwired: 1 out]
                    n263 = call <vilib>:"DAQmx Stop Task.vi"("task/channels in"=w1291, "error in"=w1290) -> ("task out"=w1289:refnum<k21>, "error out"=w1288:errorcluster)  [unwired: 12 in]
                  }
                  n264 = Multiply(x=5.0, y=w555) -> (x*y=w585:dbl)
                  n265 = To Double Precision Float(number=w558) -> (double precision float=w584:dbl)
                  n266 = Divide(x=w585, y=w584) -> (x/y=w583:dbl)
                  n267 = Reciprocal(x=w555) -> (1/x=w518:dbl)
                  n268 = To Long Integer(number=w583) -> (32bit integer=w524:i32)
                  n269 = call <vilib>:"DAQmx Clear Task.vi"("task in"=w594, "error in"=w593) -> ()  [unwired: 13 in, 1 out]
                  n270 = Obtain Queue(name (unnamed)="ch0" ("이름(이름없음)"), element data type=w523) -> (queue out=w582:refnum<queue>, error out=w581:errorcluster)  [unwired: 3 in, 1 out]
                  n271 = Obtain Queue(name (unnamed)="ch1" ("이름(이름없음)"), element data type=w523) -> (queue out=w578:refnum<queue>, error out=w577:errorcluster)  [unwired: 3 in, 1 out]
                  n272 = Obtain Queue(name (unnamed)="ch2" ("이름(이름없음)"), element data type=w523) -> (queue out=w574:refnum<queue>, error out=w573:errorcluster)  [unwired: 3 in, 1 out]
                  n273 = Obtain Queue(name (unnamed)="ch3" ("이름(이름없음)"), element data type=w523) -> (queue out=w572:refnum<queue>, error out=w571:errorcluster)  [unwired: 3 in, 1 out]
                  n274 = Obtain Queue(name (unnamed)="ch4" ("이름(이름없음)"), element data type=w523) -> (queue out=w566:refnum<queue>, error out=w565:errorcluster)  [unwired: 3 in, 1 out]
                  n275 = Obtain Queue(name (unnamed)="ch5" ("이름(이름없음)"), element data type=w523) -> (queue out=w564:refnum<queue>, error out=w563:errorcluster)  [unwired: 3 in, 1 out]
                  n276 = Obtain Queue(name (unnamed)="ch6" ("이름(이름없음)"), element data type=w523) -> (queue out=w562:refnum<queue>, error out=w561:errorcluster)  [unwired: 3 in, 1 out]
                  n277 = Obtain Queue(name (unnamed)="ch7" ("이름(이름없음)"), element data type=w523) -> (queue out=w560:refnum<queue>, error out=w559:errorcluster)  [unwired: 3 in, 1 out]
                  n278 = for {
                    N: w524 -> [_]
                    tunnel: w588 -> [w1286]
                    tunnel: w587 -> [w1285]
                    tunnel: [w1284] -> w591
                    tunnel: [w1283] -> w592
                    tunnel: w582 -> [w1282]
                    tunnel: w581 -> [w1281]
                    tunnel: w578 -> [w1280]
                    tunnel: w577 -> [w1279]
                    tunnel: w574 -> [w1278]
                    tunnel: w573 -> [w1277]
                    tunnel: w572 -> [w1276]
                    tunnel: w571 -> [w1275]
                    tunnel: w566 -> [w1274]
                    tunnel: w565 -> [w1273]
                    tunnel: w564 -> [w1272]
                    tunnel: w563 -> [w1271]
                    tunnel: w562 -> [w1270]
                    tunnel: w561 -> [w1269]
                    tunnel: w560 -> [w1268]
                    tunnel: w559 -> [w1267]
                    tunnel: w558 -> [w1257]
                    n279 = call-poly <vilib>:"DAQmx Read.vi"("task/channels in"=w1286, "number of samples per channel"=w1257, "error in"=w1285) -> ("task out"=w1284:refnum<k21>, "data"=w1258:waveform(dbl)[], "error out"=w1283:errorcluster)  [unwired: 10 out]
                    n280 = Index Array(array=w1258) -> (element #1=w1259:waveform(dbl), element #2=w1260:waveform(dbl), element #3=w1261:waveform(dbl), element #4=w1262:waveform(dbl), element #5=w1263:waveform(dbl), element #6=w1264:waveform(dbl), element #7=w1265:waveform(dbl), element #8=w1266:waveform(dbl))  [unwired: 8 in]
                    n281 = Enqueue Element(queue=w1270, element=w1265, error in (no error)=w1269) -> ()  [unwired: 1 in, 3 out]
                    n282 = Enqueue Element(queue=w1268, element=w1266, error in (no error)=w1267) -> ()  [unwired: 1 in, 3 out]
                    n283 = Enqueue Element(queue=w1278, element=w1261, error in (no error)=w1277) -> ()  [unwired: 1 in, 3 out]
                    n284 = Enqueue Element(queue=w1276, element=w1262, error in (no error)=w1275) -> ()  [unwired: 1 in, 3 out]
                    n285 = Enqueue Element(queue=w1274, element=w1263, error in (no error)=w1273) -> ()  [unwired: 1 in, 3 out]
                    n286 = Enqueue Element(queue=w1272, element=w1264, error in (no error)=w1271) -> ()  [unwired: 1 in, 3 out]
                    n287 = Enqueue Element(queue=w1282, element=w1259, error in (no error)=w1281) -> ()  [unwired: 1 in, 3 out]
                    n288 = Enqueue Element(queue=w1280, element=w1260, error in (no error)=w1279) -> ()  [unwired: 1 in, 3 out]
                  }
                  n289 = local read "Coefficient2_bit0"() -> (w522:dbl[])
                  n290 = local read "Coefficient2_bit1"() -> (w521:dbl[])
                  n291 = local read "MovingAverage_Coefficient"() -> (w520:dbl[])
                  n292 = local read "Target code"() -> (w519:dbl[])
                  n293 = call <vilib>:"DAQmx Stop Task.vi"("task/channels in"=w591, "error in"=w592) -> ("task out"=w590:refnum<k21>, "error out"=w589:errorcluster)  [unwired: 12 out]
                  n294 = call <vilib>:"DAQmx Clear Task.vi"("task in"=w590, "error in"=w589) -> ()  [unwired: 14 out]
                  n295 = flat-sequence {
                    tunnel: w523 -> [w1187]
                    tunnel: w522 -> [w1185]
                    tunnel: w521 -> [w1184]
                    tunnel: w524 -> [w1182]
                    tunnel: w520 -> [w1180]
                    tunnel: [w1181] -> w557
                    tunnel: [w1180] -> w556
                    tunnel: w518 -> [w1179]
                    tunnel: [w1179] -> w554
                    tunnel: w519 -> [w1178]
                    tunnel: [w1178] -> w553
                    tunnel: w502 -> [w1177]
                    tunnel: [w1177] -> w509
                    tunnel: w557 -> [w1209]
                    tunnel: w556 -> [w1251]
                    tunnel: w554 -> [w1218]
                    tunnel: [w1216] -> w517
                    tunnel: w553 -> [w1215]
                    tunnel: w509 -> [w1212]
                    frame #0 {
                      # "Cross correlation for bit 0 and bit 1"
                      n296 = Obtain Queue(name (unnamed)="ch0" ("이름(이름없음)"), element data type=w1187) -> (queue out=w1191:refnum<queue>, error out=w1190:errorcluster)  [unwired: 3 in, 1 out]
                      n297 = for {
                        N: w1182 -> [_]
                        tunnel: w1191 -> [w1208]
                        tunnel: w1190 -> [w1207]
                        tunnel: [w1206] -> w1189
                        tunnel: [w1205] -> w1188
                        tunnel: w1185 -> [w1195]
                        tunnel: w1184 -> [w1194]
                        tunnel: [w1192] -> w1183 mode=indexing
                        w1193 = TRUE ("init/cont (init:F)")
                        # "Whitening"
                        # "Queue\nget"
                        n298 = Dequeue Element(queue=w1208, error in (no error)=w1207) -> (queue out=w1206:refnum<queue>, element=w1200:waveform(dbl), error out=w1205:errorcluster)  [unwired: 2 out]
                        n299 = Unbundle By Name(w1200) -> ("Y"=w1199:dbl[])
                        n300 = Unbundle By Name(w1200) -> ("Y"=w1198:dbl[])
                        n301 = call-poly <vilib>:"FIR Filter.vi"("init/cont (init:F)"=w1193, "FIR Coefficients"=w1195, "X"=w1199) -> ("Filtered X"=w1204:dbl[])  [unwired: 1 in, 1 out]
                        n302 = call-poly <vilib>:"FIR Filter.vi"("init/cont (init:F)"=w1193, "FIR Coefficients"=w1194, "X"=w1198) -> ("Filtered X"=w1203:dbl[])  [unwired: 1 in, 1 out]
                        n303 = call "Envelope(SubVI).vi"("x"=w1204) -> ("Y"=w1202:dbl[])
                        n304 = call "Envelope(SubVI).vi"("x"=w1203) -> ("Y"=w1201:dbl[])
                        n305 = Square(x=w1202) -> (x^2=w1197:dbl[])
                        n306 = Square(x=w1201) -> (x^2=w1196:dbl[])
                        n307 = Subtract(x=w1197, y=w1196) -> (x-y=w1192:dbl[])
                      }
                      n308 = Release Queue(queue=w1189, error in (no error)=w1188) -> ()  [unwired: 1 in, 3 out]
                      n309 = call "2Dto1D(SubVI).vi"("X1"=w1183) -> ("Y1"=w1181:dbl[])
                    }
                    frame #1 {
                      w1234 = 75 ("width")
                      # "Peak / Valley detection, Code decision, Arrival time save"
                      # "Threshold estimation"
                      # "Decision"
                      n310 = call-poly <vilib>:"FIR Filter.vi"("FIR Coefficients"=w1251, "X"=w1209) -> ("Filtered X"=w1252:dbl[])  [unwired: 2 in, 1 out]
                      n311 = Array Max & Min(array=w1252) -> (max value=w1214:dbl, min value=w1213:dbl)  [unwired: 2 out]
                      n312 = Add(x=w1212, y=w1214) -> (x+y=w1210:dbl)
                      n313 = Subtract(x=w1213, y=w1212) -> (x-y=w1211:dbl)
                      n314 = call <vilib>:"Peak Detector.vi"("peaks/valleys"=enum32{"Peaks", "Valleys"}."Peaks", "width"=w1234, "threshold"=w1210, "X"=w1209) -> ("Amplitudes"=w1236:dbl[], "Locations"=w1233:dbl[], "# found"=w1237:i32)  [unwired: 3 in, 2 out]
                      n315 = call <vilib>:"Peak Detector.vi"("peaks/valleys"=enum32{"Peaks", "Valleys"}."Valleys", "width"=w1234, "threshold"=w1211, "X"=w1209) -> ("Amplitudes"=w1235:dbl[], "Locations"=w1232:dbl[])  [unwired: 3 in, 3 out]
                      n316 = Less Than 0?(x=w1236) -> (x < 0?=w1238:bool[])
                      n317 = Less Than 0?(x=w1235) -> (x < 0?=w1240:bool[])
                      n318 = Boolean To (0,1)(Boolean=w1238) -> (0, 1=w1248:i16[])
                      n319 = Boolean To (0,1)(Boolean=w1240) -> (0, 1=w1241:i16[])
                      n320 = To Double Precision Float(number=w1248) -> (double precision float=w1239:dbl[])
                      n321 = To Double Precision Float(number=w1241) -> (double precision float=w1242:dbl[])
                      n322 = Build Array(w1233, w1239) -> (w1244:dbl[][])
                      n323 = Build Array(w1232, w1242) -> (w1243:dbl[][])
                      n324 = Insert Into Array(array=w1244, index (col)=w1237, new element=w1243) -> (w1245:dbl[][])  [unwired: 1 in]
                      n325 = call "Sort 2D Array.vim"("index"=0, "dimension to index (column)"=enum16{"column", "row"}."row", "2D array"=w1245) -> ("sorted 2D array"=w1223:dbl[][])  [unwired: 7 in, 1 out]
                      n326 = Index Array(array=w1223) -> (element #1=w1219:dbl[], element #2=w1222:dbl[])  [unwired: 4 in]
                      n327 = Multiply(x=w1219, y=w1218) -> (x*y=w1217:dbl[])
                      n328 = Equal?(x=w1222, y=w1215) -> (x = y?=w1231:bool[])
                      n329 = Boolean Array To Number(Boolean array=w1231) -> (number=w1230:u32)
                      n330 = Array Size(array=w1215) -> (size(s)=w1227:i32)
                      n331 = To Double Precision Float(number=w1227) -> (double precision float=w1226:dbl)
                      n332 = Power Of X(1:2.0 ("x"), 2:w1226) -> (0:w1225:dbl)
                      n333 = Decrement(x=w1225) -> (x-1=w1229:dbl)
                      n334 = To Unsigned Long Integer(number=w1229) -> (unsigned 32bit integer=w1224:u32)
                      n335 = Equal?(x=w1230, y=w1224) -> (x = y?=w1221:bool)
                      n336 = case shown="참" w1221 {
                        tunnel: w1217 -> [_ w1256]
                        tunnel: dbl[] [inf, inf, inf, inf, inf, inf, inf, inf] -> [w1253 w1255]
                        tunnel: [w1253 w1254] -> w1216
                        frame False {
                        }
                        frame True {
                          n337 = Replace Array Subset(array=w1255, new element=w1256) -> (w1254:dbl[])  [unwired: 1 in]
                        }
                      }
                    }
                  }
                  n338 = flat-sequence {
                    tunnel: w523 -> [w947]
                    tunnel: w522 -> [w945]
                    tunnel: w521 -> [w944]
                    tunnel: w524 -> [w942]
                    tunnel: w520 -> [w940]
                    tunnel: [w941] -> w544
                    tunnel: [w940] -> w543
                    tunnel: w518 -> [w939]
                    tunnel: [w939] -> w542
                    tunnel: w519 -> [w938]
                    tunnel: [w938] -> w541
                    tunnel: w502 -> [w937]
                    tunnel: [w937] -> w506
                    tunnel: w544 -> [w974]
                    tunnel: w543 -> [w1011]
                    tunnel: w542 -> [w978]
                    tunnel: [w976] -> w514
                    tunnel: w541 -> [w975]
                    tunnel: w506 -> [w971]
                    frame #0 {
                      n339 = Obtain Queue(name (unnamed)="ch3" ("이름(이름없음)"), element data type=w947) -> (queue out=w951:refnum<queue>, error out=w950:errorcluster)  [unwired: 3 in, 1 out]
                      n340 = for {
                        N: w942 -> [_]
                        tunnel: w951 -> [w968]
                        tunnel: w950 -> [w967]
                        tunnel: [w966] -> w949
                        tunnel: [w965] -> w948
                        tunnel: w945 -> [w955]
                        tunnel: w944 -> [w954]
                        tunnel: [w952] -> w943 mode=indexing
                        w953 = TRUE ("init/cont (init:F)")
                        n341 = Dequeue Element(queue=w968, error in (no error)=w967) -> (queue out=w966:refnum<queue>, element=w960:waveform(dbl), error out=w965:errorcluster)  [unwired: 2 out]
                        n342 = Unbundle By Name(w960) -> ("Y"=w959:dbl[])
                        n343 = Unbundle By Name(w960) -> ("Y"=w958:dbl[])
                        n344 = call-poly <vilib>:"FIR Filter.vi"("init/cont (init:F)"=w953, "FIR Coefficients"=w955, "X"=w959) -> ("Filtered X"=w964:dbl[])  [unwired: 1 in, 1 out]
                        n345 = call-poly <vilib>:"FIR Filter.vi"("init/cont (init:F)"=w953, "FIR Coefficients"=w954, "X"=w958) -> ("Filtered X"=w963:dbl[])  [unwired: 1 in, 1 out]
                        n346 = call "Envelope(SubVI).vi"("x"=w964) -> ("Y"=w962:dbl[])
                        n347 = call "Envelope(SubVI).vi"("x"=w963) -> ("Y"=w961:dbl[])
                        n348 = Square(x=w962) -> (x^2=w957:dbl[])
                        n349 = Square(x=w961) -> (x^2=w956:dbl[])
                        n350 = Subtract(x=w957, y=w956) -> (x-y=w952:dbl[])
                      }
                      n351 = Release Queue(queue=w949, error in (no error)=w948) -> ()  [unwired: 1 in, 3 out]
                      n352 = call "2Dto1D(SubVI).vi"("X1"=w943) -> ("Y1"=w941:dbl[])
                    }
                    frame #1 {
                      w994 = 75 ("width")
                      # "Sort"
                      # "Decision"
                      n353 = call-poly <vilib>:"FIR Filter.vi"("FIR Coefficients"=w1011, "X"=w974) -> ("Filtered X"=w1012:dbl[])  [unwired: 2 in, 1 out]
                      n354 = Array Max & Min(array=w1012) -> (max value=w973:dbl, min value=w972:dbl)  [unwired: 2 out]
                      n355 = Add(x=w971, y=w973) -> (x+y=w970:dbl)
                      n356 = Subtract(x=w972, y=w971) -> (x-y=w969:dbl)
                      n357 = call <vilib>:"Peak Detector.vi"("peaks/valleys"=enum32{"Peaks", "Valleys"}."Peaks", "width"=w994, "threshold"=w970, "X"=w974) -> ("Amplitudes"=w996:dbl[], "Locations"=w993:dbl[], "# found"=w997:i32)  [unwired: 3 in, 2 out]
                      n358 = call <vilib>:"Peak Detector.vi"("peaks/valleys"=enum32{"Peaks", "Valleys"}."Valleys", "width"=w994, "threshold"=w969, "X"=w974) -> ("Amplitudes"=w995:dbl[], "Locations"=w992:dbl[])  [unwired: 3 in, 3 out]
                      n359 = Less Than 0?(x=w996) -> (x < 0?=w998:bool[])
                      n360 = Less Than 0?(x=w995) -> (x < 0?=w1000:bool[])
                      n361 = Boolean To (0,1)(Boolean=w998) -> (0, 1=w1008:i16[])
                      n362 = Boolean To (0,1)(Boolean=w1000) -> (0, 1=w1001:i16[])
                      n363 = To Double Precision Float(number=w1008) -> (double precision float=w999:dbl[])
                      n364 = To Double Precision Float(number=w1001) -> (double precision float=w1002:dbl[])
                      n365 = Build Array(w993, w999) -> (w1004:dbl[][])
                      n366 = Build Array(w992, w1002) -> (w1003:dbl[][])
                      n367 = Insert Into Array(array=w1004, index (col)=w997, new element=w1003) -> (w1005:dbl[][])  [unwired: 1 in]
                      n368 = call "Sort 2D Array.vim"("index"=0, "dimension to index (column)"=enum16{"column", "row"}."row", "2D array"=w1005) -> ("sorted 2D array"=w983:dbl[][])  [unwired: 7 in, 1 out]
                      n369 = Index Array(array=w983) -> (element #1=w979:dbl[], element #2=w982:dbl[])  [unwired: 4 in]
                      n370 = Multiply(x=w979, y=w978) -> (x*y=w977:dbl[])
                      n371 = Equal?(x=w982, y=w975) -> (x = y?=w991:bool[])
                      n372 = Boolean Array To Number(Boolean array=w991) -> (number=w990:u32)
                      n373 = Array Size(array=w975) -> (size(s)=w987:i32)
                      n374 = To Double Precision Float(number=w987) -> (double precision float=w986:dbl)
                      n375 = Power Of X(1:2.0 ("x"), 2:w986) -> (0:w985:dbl)
                      n376 = Decrement(x=w985) -> (x-1=w989:dbl)
                      n377 = To Unsigned Long Integer(number=w989) -> (unsigned 32bit integer=w984:u32)
                      n378 = Equal?(x=w990, y=w984) -> (x = y?=w981:bool)
                      n379 = case shown="참" w981 {
                        tunnel: w977 -> [_ w1016]
                        tunnel: dbl[] [inf, inf, inf, inf, inf, inf, inf, inf] -> [w1013 w1015]
                        tunnel: [w1013 w1014] -> w976
                        frame False {
                        }
                        frame True {
                          n380 = Replace Array Subset(array=w1015, new element=w1016) -> (w1014:dbl[])  [unwired: 1 in]
                        }
                      }
                    }
                  }
                  n381 = flat-sequence {
                    tunnel: w523 -> [w1107]
                    tunnel: [w1099] -> _
                    tunnel: [w1098] -> _
                    tunnel: w524 -> [w1104]
                    tunnel: w520 -> [w1102]
                    tunnel: [w1103] -> w552
                    tunnel: [w1102] -> w551
                    tunnel: w518 -> [w1101]
                    tunnel: [w1101] -> w550
                    tunnel: w519 -> [w1100]
                    tunnel: [w1100] -> w549
                    tunnel: w522 -> [w1099]
                    tunnel: w521 -> [w1098]
                    tunnel: w502 -> [w1097]
                    tunnel: [w1097] -> w508
                    tunnel: w552 -> [w1134]
                    tunnel: w551 -> [w1171]
                    tunnel: w550 -> [w1138]
                    tunnel: [w1136] -> w516
                    tunnel: w549 -> [w1135]
                    tunnel: w508 -> [w1131]
                    frame #0 {
                      n382 = Obtain Queue(name (unnamed)="ch1" ("이름(이름없음)"), element data type=w1107) -> (queue out=w1111:refnum<queue>, error out=w1110:errorcluster)  [unwired: 3 in, 1 out]
                      n383 = for {
                        N: w1104 -> [_]
                        tunnel: w1111 -> [w1128]
                        tunnel: w1110 -> [w1127]
                        tunnel: [w1126] -> w1109
                        tunnel: [w1125] -> w1108
                        tunnel: w1099 -> [w1115]
                        tunnel: w1098 -> [w1114]
                        tunnel: [w1112] -> w1105 mode=indexing
                        w1113 = TRUE ("init/cont (init:F)")
                        n384 = Dequeue Element(queue=w1128, error in (no error)=w1127) -> (queue out=w1126:refnum<queue>, element=w1120:waveform(dbl), error out=w1125:errorcluster)  [unwired: 2 out]
                        n385 = Unbundle By Name(w1120) -> ("Y"=w1119:dbl[])
                        n386 = Unbundle By Name(w1120) -> ("Y"=w1118:dbl[])
                        n387 = call-poly <vilib>:"FIR Filter.vi"("init/cont (init:F)"=w1113, "FIR Coefficients"=w1115, "X"=w1119) -> ("Filtered X"=w1124:dbl[])  [unwired: 1 in, 1 out]
                        n388 = call-poly <vilib>:"FIR Filter.vi"("init/cont (init:F)"=w1113, "FIR Coefficients"=w1114, "X"=w1118) -> ("Filtered X"=w1123:dbl[])  [unwired: 1 in, 1 out]
                        n389 = call "Envelope(SubVI).vi"("x"=w1124) -> ("Y"=w1122:dbl[])
                        n390 = call "Envelope(SubVI).vi"("x"=w1123) -> ("Y"=w1121:dbl[])
                        n391 = Square(x=w1122) -> (x^2=w1117:dbl[])
                        n392 = Square(x=w1121) -> (x^2=w1116:dbl[])
                        n393 = Subtract(x=w1117, y=w1116) -> (x-y=w1112:dbl[])
                      }
                      n394 = Release Queue(queue=w1109, error in (no error)=w1108) -> ()  [unwired: 1 in, 3 out]
                      n395 = call "2Dto1D(SubVI).vi"("X1"=w1105) -> ("Y1"=w1103:dbl[])
                    }
                    frame #1 {
                      w1154 = 75 ("width")
                      # "Sort"
                      # "Decision"
                      n396 = call-poly <vilib>:"FIR Filter.vi"("FIR Coefficients"=w1171, "X"=w1134) -> ("Filtered X"=w1172:dbl[])  [unwired: 2 in, 1 out]
                      n397 = Array Max & Min(array=w1172) -> (max value=w1133:dbl, min value=w1132:dbl)  [unwired: 2 out]
                      n398 = Add(x=w1131, y=w1133) -> (x+y=w1130:dbl)
                      n399 = Subtract(x=w1132, y=w1131) -> (x-y=w1129:dbl)
                      n400 = call <vilib>:"Peak Detector.vi"("peaks/valleys"=enum32{"Peaks", "Valleys"}."Peaks", "width"=w1154, "threshold"=w1130, "X"=w1134) -> ("Amplitudes"=w1156:dbl[], "Locations"=w1153:dbl[], "# found"=w1157:i32)  [unwired: 3 in, 2 out]
                      n401 = call <vilib>:"Peak Detector.vi"("peaks/valleys"=enum32{"Peaks", "Valleys"}."Valleys", "width"=w1154, "threshold"=w1129, "X"=w1134) -> ("Amplitudes"=w1155:dbl[], "Locations"=w1152:dbl[])  [unwired: 3 in, 3 out]
                      n402 = Less Than 0?(x=w1156) -> (x < 0?=w1158:bool[])
                      n403 = Less Than 0?(x=w1155) -> (x < 0?=w1160:bool[])
                      n404 = Boolean To (0,1)(Boolean=w1158) -> (0, 1=w1168:i16[])
                      n405 = Boolean To (0,1)(Boolean=w1160) -> (0, 1=w1161:i16[])
                      n406 = To Double Precision Float(number=w1168) -> (double precision float=w1159:dbl[])
                      n407 = To Double Precision Float(number=w1161) -> (double precision float=w1162:dbl[])
                      n408 = Build Array(w1153, w1159) -> (w1164:dbl[][])
                      n409 = Build Array(w1152, w1162) -> (w1163:dbl[][])
                      n410 = Insert Into Array(array=w1164, index (col)=w1157, new element=w1163) -> (w1165:dbl[][])  [unwired: 1 in]
                      n411 = call "Sort 2D Array.vim"("index"=0, "dimension to index (column)"=enum16{"column", "row"}."row", "2D array"=w1165) -> ("sorted 2D array"=w1143:dbl[][])  [unwired: 7 in, 1 out]
                      n412 = Index Array(array=w1143) -> (element #1=w1139:dbl[], element #2=w1142:dbl[])  [unwired: 4 in]
                      n413 = Multiply(x=w1139, y=w1138) -> (x*y=w1137:dbl[])
                      n414 = Equal?(x=w1142, y=w1135) -> (x = y?=w1151:bool[])
                      n415 = Boolean Array To Number(Boolean array=w1151) -> (number=w1150:u32)
                      n416 = Array Size(array=w1135) -> (size(s)=w1147:i32)
                      n417 = To Double Precision Float(number=w1147) -> (double precision float=w1146:dbl)
                      n418 = Power Of X(1:2.0 ("x"), 2:w1146) -> (0:w1145:dbl)
                      n419 = Decrement(x=w1145) -> (x-1=w1149:dbl)
                      n420 = To Unsigned Long Integer(number=w1149) -> (unsigned 32bit integer=w1144:u32)
                      n421 = Equal?(x=w1150, y=w1144) -> (x = y?=w1141:bool)
                      n422 = case shown="참" w1141 {
                        tunnel: w1137 -> [_ w1176]
                        tunnel: dbl[] [inf, inf, inf, inf, inf, inf, inf, inf] -> [w1173 w1175]
                        tunnel: [w1173 w1174] -> w1136
                        frame False {
                        }
                        frame True {
                          n423 = Replace Array Subset(array=w1175, new element=w1176) -> (w1174:dbl[])  [unwired: 1 in]
                        }
                      }
                    }
                  }
                  n424 = flat-sequence {
                    tunnel: w523 -> [w1027]
                    tunnel: w522 -> [w1025]
                    tunnel: w521 -> [w1024]
                    tunnel: w524 -> [w1022]
                    tunnel: w520 -> [w1020]
                    tunnel: [w1021] -> w548
                    tunnel: [w1020] -> w547
                    tunnel: w518 -> [w1019]
                    tunnel: [w1019] -> w546
                    tunnel: w519 -> [w1018]
                    tunnel: [w1018] -> w545
                    tunnel: w502 -> [w1017]
                    tunnel: [w1017] -> w507
                    tunnel: w548 -> [w1054]
                    tunnel: w547 -> [w1091]
                    tunnel: w546 -> [w1058]
                    tunnel: [w1056] -> w515
                    tunnel: w545 -> [w1055]
                    tunnel: w507 -> [w1051]
                    frame #0 {
                      n425 = Obtain Queue(name (unnamed)="ch2" ("이름(이름없음)"), element data type=w1027) -> (queue out=w1031:refnum<queue>, error out=w1030:errorcluster)  [unwired: 3 in, 1 out]
                      n426 = for {
                        N: w1022 -> [_]
                        tunnel: w1031 -> [w1048]
                        tunnel: w1030 -> [w1047]
                        tunnel: [w1046] -> w1029
                        tunnel: [w1045] -> w1028
                        tunnel: w1025 -> [w1035]
                        tunnel: w1024 -> [w1034]
                        tunnel: [w1032] -> w1023 mode=indexing
                        w1033 = TRUE ("init/cont (init:F)")
                        n427 = Dequeue Element(queue=w1048, error in (no error)=w1047) -> (queue out=w1046:refnum<queue>, element=w1040:waveform(dbl), error out=w1045:errorcluster)  [unwired: 2 out]
                        n428 = Unbundle By Name(w1040) -> ("Y"=w1039:dbl[])
                        n429 = Unbundle By Name(w1040) -> ("Y"=w1038:dbl[])
                        n430 = call-poly <vilib>:"FIR Filter.vi"("init/cont (init:F)"=w1033, "FIR Coefficients"=w1035, "X"=w1039) -> ("Filtered X"=w1044:dbl[])  [unwired: 1 in, 1 out]
                        n431 = call-poly <vilib>:"FIR Filter.vi"("init/cont (init:F)"=w1033, "FIR Coefficients"=w1034, "X"=w1038) -> ("Filtered X"=w1043:dbl[])  [unwired: 1 in, 1 out]
                        n432 = call "Envelope(SubVI).vi"("x"=w1044) -> ("Y"=w1042:dbl[])
                        n433 = call "Envelope(SubVI).vi"("x"=w1043) -> ("Y"=w1041:dbl[])
                        n434 = Square(x=w1042) -> (x^2=w1037:dbl[])
                        n435 = Square(x=w1041) -> (x^2=w1036:dbl[])
                        n436 = Subtract(x=w1037, y=w1036) -> (x-y=w1032:dbl[])
                      }
                      n437 = Release Queue(queue=w1029, error in (no error)=w1028) -> ()  [unwired: 1 in, 3 out]
                      n438 = call "2Dto1D(SubVI).vi"("X1"=w1023) -> ("Y1"=w1021:dbl[])
                    }
                    frame #1 {
                      w1074 = 75 ("width")
                      # "Sort"
                      # "Decision"
                      n439 = call-poly <vilib>:"FIR Filter.vi"("FIR Coefficients"=w1091, "X"=w1054) -> ("Filtered X"=w1092:dbl[])  [unwired: 2 in, 1 out]
                      n440 = Array Max & Min(array=w1092) -> (max value=w1053:dbl, min value=w1052:dbl)  [unwired: 2 out]
                      n441 = Add(x=w1051, y=w1053) -> (x+y=w1050:dbl)
                      n442 = Subtract(x=w1052, y=w1051) -> (x-y=w1049:dbl)
                      n443 = call <vilib>:"Peak Detector.vi"("peaks/valleys"=enum32{"Peaks", "Valleys"}."Peaks", "width"=w1074, "threshold"=w1050, "X"=w1054) -> ("Amplitudes"=w1076:dbl[], "Locations"=w1073:dbl[], "# found"=w1077:i32)  [unwired: 3 in, 2 out]
                      n444 = call <vilib>:"Peak Detector.vi"("peaks/valleys"=enum32{"Peaks", "Valleys"}."Valleys", "width"=w1074, "threshold"=w1049, "X"=w1054) -> ("Amplitudes"=w1075:dbl[], "Locations"=w1072:dbl[])  [unwired: 3 in, 3 out]
                      n445 = Less Than 0?(x=w1076) -> (x < 0?=w1078:bool[])
                      n446 = Less Than 0?(x=w1075) -> (x < 0?=w1080:bool[])
                      n447 = Boolean To (0,1)(Boolean=w1078) -> (0, 1=w1088:i16[])
                      n448 = Boolean To (0,1)(Boolean=w1080) -> (0, 1=w1081:i16[])
                      n449 = To Double Precision Float(number=w1088) -> (double precision float=w1079:dbl[])
                      n450 = To Double Precision Float(number=w1081) -> (double precision float=w1082:dbl[])
                      n451 = Build Array(w1073, w1079) -> (w1084:dbl[][])
                      n452 = Build Array(w1072, w1082) -> (w1083:dbl[][])
                      n453 = Insert Into Array(array=w1084, index (col)=w1077, new element=w1083) -> (w1085:dbl[][])  [unwired: 1 in]
                      n454 = call "Sort 2D Array.vim"("index"=0, "dimension to index (column)"=enum16{"column", "row"}."row", "2D array"=w1085) -> ("sorted 2D array"=w1063:dbl[][])  [unwired: 7 in, 1 out]
                      n455 = Index Array(array=w1063) -> (element #1=w1059:dbl[], element #2=w1062:dbl[])  [unwired: 4 in]
                      n456 = Multiply(x=w1059, y=w1058) -> (x*y=w1057:dbl[])
                      n457 = Equal?(x=w1062, y=w1055) -> (x = y?=w1071:bool[])
                      n458 = Boolean Array To Number(Boolean array=w1071) -> (number=w1070:u32)
                      n459 = Array Size(array=w1055) -> (size(s)=w1067:i32)
                      n460 = To Double Precision Float(number=w1067) -> (double precision float=w1066:dbl)
                      n461 = Power Of X(1:2.0 ("x"), 2:w1066) -> (0:w1065:dbl)
                      n462 = Decrement(x=w1065) -> (x-1=w1069:dbl)
                      n463 = To Unsigned Long Integer(number=w1069) -> (unsigned 32bit integer=w1064:u32)
                      n464 = Equal?(x=w1070, y=w1064) -> (x = y?=w1061:bool)
                      n465 = case shown="참" w1061 {
                        tunnel: w1057 -> [_ w1096]
                        tunnel: dbl[] [inf, inf, inf, inf, inf, inf, inf, inf] -> [w1093 w1095]
                        tunnel: [w1093 w1094] -> w1056
                        frame False {
                        }
                        frame True {
                          n466 = Replace Array Subset(array=w1095, new element=w1096) -> (w1094:dbl[])  [unwired: 1 in]
                        }
                      }
                    }
                  }
                  n467 = flat-sequence {
                    tunnel: w523 -> [w867]
                    tunnel: w522 -> [w865]
                    tunnel: w521 -> [w864]
                    tunnel: w524 -> [w862]
                    tunnel: w520 -> [w860]
                    tunnel: [w861] -> w540
                    tunnel: [w860] -> w539
                    tunnel: w518 -> [w859]
                    tunnel: [w859] -> w538
                    tunnel: w519 -> [w858]
                    tunnel: [w858] -> w537
                    tunnel: w502 -> [w857]
                    tunnel: [w857] -> w505
                    tunnel: w540 -> [w894]
                    tunnel: w539 -> [w931]
                    tunnel: w538 -> [w898]
                    tunnel: [w896] -> w513
                    tunnel: w537 -> [w895]
                    tunnel: w505 -> [w889]
                    frame #0 {
                      n468 = Obtain Queue(name (unnamed)="ch4" ("이름(이름없음)"), element data type=w867) -> (queue out=w871:refnum<queue>, error out=w870:errorcluster)  [unwired: 3 in, 1 out]
                      n469 = for {
                        N: w862 -> [_]
                        tunnel: w871 -> [w888]
                        tunnel: w870 -> [w887]
                        tunnel: [w886] -> w869
                        tunnel: [w885] -> w868
                        tunnel: w865 -> [w875]
                        tunnel: w864 -> [w874]
                        tunnel: [w872] -> w863 mode=indexing
                        w873 = TRUE ("init/cont (init:F)")
                        n470 = Dequeue Element(queue=w888, error in (no error)=w887) -> (queue out=w886:refnum<queue>, element=w880:waveform(dbl), error out=w885:errorcluster)  [unwired: 2 out]
                        n471 = Unbundle By Name(w880) -> ("Y"=w879:dbl[])
                        n472 = Unbundle By Name(w880) -> ("Y"=w878:dbl[])
                        n473 = call-poly <vilib>:"FIR Filter.vi"("init/cont (init:F)"=w873, "FIR Coefficients"=w875, "X"=w879) -> ("Filtered X"=w884:dbl[])  [unwired: 1 in, 1 out]
                        n474 = call-poly <vilib>:"FIR Filter.vi"("init/cont (init:F)"=w873, "FIR Coefficients"=w874, "X"=w878) -> ("Filtered X"=w883:dbl[])  [unwired: 1 in, 1 out]
                        n475 = call "Envelope(SubVI).vi"("x"=w884) -> ("Y"=w882:dbl[])
                        n476 = call "Envelope(SubVI).vi"("x"=w883) -> ("Y"=w881:dbl[])
                        n477 = Square(x=w882) -> (x^2=w877:dbl[])
                        n478 = Square(x=w881) -> (x^2=w876:dbl[])
                        n479 = Subtract(x=w877, y=w876) -> (x-y=w872:dbl[])
                      }
                      n480 = Release Queue(queue=w869, error in (no error)=w868) -> ()  [unwired: 1 in, 3 out]
                      n481 = call "2Dto1D(SubVI).vi"("X1"=w863) -> ("Y1"=w861:dbl[])
                    }
                    frame #1 {
                      w914 = 75 ("width")
                      # "Sort"
                      # "Decision"
                      n482 = call-poly <vilib>:"FIR Filter.vi"("FIR Coefficients"=w931, "X"=w894) -> ("Filtered X"=w932:dbl[])  [unwired: 2 in, 1 out]
                      n483 = Array Max & Min(array=w932) -> (max value=w893:dbl, min value=w892:dbl)  [unwired: 2 out]
                      n484 = Add(x=w889, y=w893) -> (x+y=w891:dbl)
                      n485 = Subtract(x=w892, y=w889) -> (x-y=w890:dbl)
                      n486 = call <vilib>:"Peak Detector.vi"("peaks/valleys"=enum32{"Peaks", "Valleys"}."Peaks", "width"=w914, "threshold"=w891, "X"=w894) -> ("Amplitudes"=w916:dbl[], "Locations"=w913:dbl[], "# found"=w917:i32)  [unwired: 3 in, 2 out]
                      n487 = call <vilib>:"Peak Detector.vi"("peaks/valleys"=enum32{"Peaks", "Valleys"}."Valleys", "width"=w914, "threshold"=w890, "X"=w894) -> ("Amplitudes"=w915:dbl[], "Locations"=w912:dbl[])  [unwired: 3 in, 3 out]
                      n488 = Less Than 0?(x=w916) -> (x < 0?=w918:bool[])
                      n489 = Less Than 0?(x=w915) -> (x < 0?=w920:bool[])
                      n490 = Boolean To (0,1)(Boolean=w918) -> (0, 1=w928:i16[])
                      n491 = Boolean To (0,1)(Boolean=w920) -> (0, 1=w921:i16[])
                      n492 = To Double Precision Float(number=w928) -> (double precision float=w919:dbl[])
                      n493 = To Double Precision Float(number=w921) -> (double precision float=w922:dbl[])
                      n494 = Build Array(w913, w919) -> (w924:dbl[][])
                      n495 = Build Array(w912, w922) -> (w923:dbl[][])
                      n496 = Insert Into Array(array=w924, index (col)=w917, new element=w923) -> (w925:dbl[][])  [unwired: 1 in]
                      n497 = call "Sort 2D Array.vim"("index"=0, "dimension to index (column)"=enum16{"column", "row"}."row", "2D array"=w925) -> ("sorted 2D array"=w903:dbl[][])  [unwired: 7 in, 1 out]
                      n498 = Index Array(array=w903) -> (element #1=w899:dbl[], element #2=w902:dbl[])  [unwired: 4 in]
                      n499 = Multiply(x=w899, y=w898) -> (x*y=w897:dbl[])
                      n500 = Equal?(x=w902, y=w895) -> (x = y?=w911:bool[])
                      n501 = Boolean Array To Number(Boolean array=w911) -> (number=w910:u32)
                      n502 = Array Size(array=w895) -> (size(s)=w907:i32)
                      n503 = To Double Precision Float(number=w907) -> (double precision float=w906:dbl)
                      n504 = Power Of X(1:2.0 ("x"), 2:w906) -> (0:w905:dbl)
                      n505 = Decrement(x=w905) -> (x-1=w909:dbl)
                      n506 = To Unsigned Long Integer(number=w909) -> (unsigned 32bit integer=w904:u32)
                      n507 = Equal?(x=w910, y=w904) -> (x = y?=w901:bool)
                      n508 = case shown="참" w901 {
                        tunnel: w897 -> [_ w936]
                        tunnel: dbl[] [inf, inf, inf, inf, inf, inf, inf, inf] -> [w933 w935]
                        tunnel: [w933 w934] -> w896
                        frame False {
                        }
                        frame True {
                          n509 = Replace Array Subset(array=w935, new element=w936) -> (w934:dbl[])  [unwired: 1 in]
                        }
                      }
                    }
                  }
                  n510 = flat-sequence {
                    tunnel: w523 -> [w787]
                    tunnel: w522 -> [w785]
                    tunnel: w521 -> [w784]
                    tunnel: [w778] -> _
                    tunnel: w520 -> [w781]
                    tunnel: [w782] -> w536
                    tunnel: [w781] -> w535
                    tunnel: w518 -> [w780]
                    tunnel: [w780] -> w534
                    tunnel: w519 -> [w779]
                    tunnel: [w779] -> w533
                    tunnel: w524 -> [w778]
                    tunnel: w502 -> [w777]
                    tunnel: [w777] -> w504
                    tunnel: w536 -> [w814]
                    tunnel: w535 -> [w851]
                    tunnel: w534 -> [w818]
                    tunnel: [w816] -> w512
                    tunnel: w533 -> [w815]
                    tunnel: w504 -> [w811]
                    frame #0 {
                      n511 = Obtain Queue(name (unnamed)="ch5" ("이름(이름없음)"), element data type=w787) -> (queue out=w791:refnum<queue>, error out=w790:errorcluster)  [unwired: 3 in, 1 out]
                      n512 = for {
                        N: w778 -> [_]
                        tunnel: w791 -> [w808]
                        tunnel: w790 -> [w807]
                        tunnel: [w806] -> w789
                        tunnel: [w805] -> w788
                        tunnel: w785 -> [w795]
                        tunnel: w784 -> [w794]
                        tunnel: [w792] -> w783 mode=indexing
                        w793 = TRUE ("init/cont (init:F)")
                        n513 = Dequeue Element(queue=w808, error in (no error)=w807) -> (queue out=w806:refnum<queue>, element=w800:waveform(dbl), error out=w805:errorcluster)  [unwired: 2 out]
                        n514 = Unbundle By Name(w800) -> ("Y"=w799:dbl[])
                        n515 = Unbundle By Name(w800) -> ("Y"=w798:dbl[])
                        n516 = call-poly <vilib>:"FIR Filter.vi"("init/cont (init:F)"=w793, "FIR Coefficients"=w795, "X"=w799) -> ("Filtered X"=w804:dbl[])  [unwired: 1 in, 1 out]
                        n517 = call-poly <vilib>:"FIR Filter.vi"("init/cont (init:F)"=w793, "FIR Coefficients"=w794, "X"=w798) -> ("Filtered X"=w803:dbl[])  [unwired: 1 in, 1 out]
                        n518 = call "Envelope(SubVI).vi"("x"=w804) -> ("Y"=w802:dbl[])
                        n519 = call "Envelope(SubVI).vi"("x"=w803) -> ("Y"=w801:dbl[])
                        n520 = Square(x=w802) -> (x^2=w797:dbl[])
                        n521 = Square(x=w801) -> (x^2=w796:dbl[])
                        n522 = Subtract(x=w797, y=w796) -> (x-y=w792:dbl[])
                      }
                      n523 = Release Queue(queue=w789, error in (no error)=w788) -> ()  [unwired: 1 in, 3 out]
                      n524 = call "2Dto1D(SubVI).vi"("X1"=w783) -> ("Y1"=w782:dbl[])
                    }
                    frame #1 {
                      w834 = 75 ("width")
                      # "Sort"
                      # "Decision"
                      n525 = call-poly <vilib>:"FIR Filter.vi"("FIR Coefficients"=w851, "X"=w814) -> ("Filtered X"=w852:dbl[])  [unwired: 2 in, 1 out]
                      n526 = Array Max & Min(array=w852) -> (max value=w813:dbl, min value=w812:dbl)  [unwired: 2 out]
                      n527 = Add(x=w811, y=w813) -> (x+y=w810:dbl)
                      n528 = Subtract(x=w812, y=w811) -> (x-y=w809:dbl)
                      n529 = call <vilib>:"Peak Detector.vi"("peaks/valleys"=enum32{"Peaks", "Valleys"}."Peaks", "width"=w834, "threshold"=w810, "X"=w814) -> ("Amplitudes"=w836:dbl[], "Locations"=w833:dbl[], "# found"=w837:i32)  [unwired: 3 in, 2 out]
                      n530 = call <vilib>:"Peak Detector.vi"("peaks/valleys"=enum32{"Peaks", "Valleys"}."Valleys", "width"=w834, "threshold"=w809, "X"=w814) -> ("Amplitudes"=w835:dbl[], "Locations"=w832:dbl[])  [unwired: 3 in, 3 out]
                      n531 = Less Than 0?(x=w836) -> (x < 0?=w838:bool[])
                      n532 = Less Than 0?(x=w835) -> (x < 0?=w840:bool[])
                      n533 = Boolean To (0,1)(Boolean=w838) -> (0, 1=w848:i16[])
                      n534 = Boolean To (0,1)(Boolean=w840) -> (0, 1=w841:i16[])
                      n535 = To Double Precision Float(number=w848) -> (double precision float=w839:dbl[])
                      n536 = To Double Precision Float(number=w841) -> (double precision float=w842:dbl[])
                      n537 = Build Array(w833, w839) -> (w844:dbl[][])
                      n538 = Build Array(w832, w842) -> (w843:dbl[][])
                      n539 = Insert Into Array(array=w844, index (col)=w837, new element=w843) -> (w845:dbl[][])  [unwired: 1 in]
                      n540 = call "Sort 2D Array.vim"("index"=0, "dimension to index (column)"=enum16{"column", "row"}."row", "2D array"=w845) -> ("sorted 2D array"=w823:dbl[][])  [unwired: 7 in, 1 out]
                      n541 = Index Array(array=w823) -> (element #1=w819:dbl[], element #2=w822:dbl[])  [unwired: 4 in]
                      n542 = Multiply(x=w819, y=w818) -> (x*y=w817:dbl[])
                      n543 = Equal?(x=w822, y=w815) -> (x = y?=w831:bool[])
                      n544 = Boolean Array To Number(Boolean array=w831) -> (number=w830:u32)
                      n545 = Array Size(array=w815) -> (size(s)=w827:i32)
                      n546 = To Double Precision Float(number=w827) -> (double precision float=w826:dbl)
                      n547 = Power Of X(1:2.0 ("x"), 2:w826) -> (0:w825:dbl)
                      n548 = Decrement(x=w825) -> (x-1=w829:dbl)
                      n549 = To Unsigned Long Integer(number=w829) -> (unsigned 32bit integer=w824:u32)
                      n550 = Equal?(x=w830, y=w824) -> (x = y?=w821:bool)
                      n551 = case shown="참" w821 {
                        tunnel: w817 -> [_ w856]
                        tunnel: dbl[] [inf, inf, inf, inf, inf, inf, inf, inf] -> [w853 w855]
                        tunnel: [w853 w854] -> w816
                        frame False {
                        }
                        frame True {
                          n552 = Replace Array Subset(array=w855, new element=w856) -> (w854:dbl[])  [unwired: 1 in]
                        }
                      }
                    }
                  }
                  n553 = flat-sequence {
                    tunnel: w523 -> [w707]
                    tunnel: w522 -> [w705]
                    tunnel: w521 -> [w704]
                    tunnel: w524 -> [w702]
                    tunnel: w520 -> [w700]
                    tunnel: [w701] -> w532
                    tunnel: [w700] -> w531
                    tunnel: w518 -> [w699]
                    tunnel: [w699] -> w530
                    tunnel: w519 -> [w698]
                    tunnel: [w698] -> w529
                    tunnel: w502 -> [w697]
                    tunnel: [w697] -> w503
                    tunnel: w532 -> [w729]
                    tunnel: w531 -> [w771]
                    tunnel: w530 -> [w738]
                    tunnel: [w736] -> w511
                    tunnel: w529 -> [w735]
                    tunnel: w503 -> [w732]
                    frame #0 {
                      n554 = Obtain Queue(name (unnamed)="ch6" ("이름(이름없음)"), element data type=w707) -> (queue out=w711:refnum<queue>, error out=w710:errorcluster)  [unwired: 3 in, 1 out]
                      n555 = for {
                        N: w702 -> [_]
                        tunnel: w711 -> [w728]
                        tunnel: w710 -> [w727]
                        tunnel: [w726] -> w709
                        tunnel: [w725] -> w708
                        tunnel: w705 -> [w715]
                        tunnel: w704 -> [w714]
                        tunnel: [w712] -> w703 mode=indexing
                        w713 = TRUE ("init/cont (init:F)")
                        n556 = Dequeue Element(queue=w728, error in (no error)=w727) -> (queue out=w726:refnum<queue>, element=w720:waveform(dbl), error out=w725:errorcluster)  [unwired: 2 out]
                        n557 = Unbundle By Name(w720) -> ("Y"=w719:dbl[])
                        n558 = Unbundle By Name(w720) -> ("Y"=w718:dbl[])
                        n559 = call-poly <vilib>:"FIR Filter.vi"("init/cont (init:F)"=w713, "FIR Coefficients"=w715, "X"=w719) -> ("Filtered X"=w724:dbl[])  [unwired: 1 in, 1 out]
                        n560 = call-poly <vilib>:"FIR Filter.vi"("init/cont (init:F)"=w713, "FIR Coefficients"=w714, "X"=w718) -> ("Filtered X"=w723:dbl[])  [unwired: 1 in, 1 out]
                        n561 = call "Envelope(SubVI).vi"("x"=w724) -> ("Y"=w722:dbl[])
                        n562 = call "Envelope(SubVI).vi"("x"=w723) -> ("Y"=w721:dbl[])
                        n563 = Square(x=w722) -> (x^2=w717:dbl[])
                        n564 = Square(x=w721) -> (x^2=w716:dbl[])
                        n565 = Subtract(x=w717, y=w716) -> (x-y=w712:dbl[])
                      }
                      n566 = Release Queue(queue=w709, error in (no error)=w708) -> ()  [unwired: 1 in, 3 out]
                      n567 = call "2Dto1D(SubVI).vi"("X1"=w703) -> ("Y1"=w701:dbl[])
                    }
                    frame #1 {
                      w754 = 75 ("width")
                      # "Sort"
                      # "Decision"
                      n568 = call-poly <vilib>:"FIR Filter.vi"("FIR Coefficients"=w771, "X"=w729) -> ("Filtered X"=w772:dbl[])  [unwired: 2 in, 1 out]
                      n569 = Array Max & Min(array=w772) -> (max value=w734:dbl, min value=w733:dbl)  [unwired: 2 out]
                      n570 = Add(x=w732, y=w734) -> (x+y=w731:dbl)
                      n571 = Subtract(x=w733, y=w732) -> (x-y=w730:dbl)
                      n572 = call <vilib>:"Peak Detector.vi"("peaks/valleys"=enum32{"Peaks", "Valleys"}."Peaks", "width"=w754, "threshold"=w731, "X"=w729) -> ("Amplitudes"=w756:dbl[], "Locations"=w753:dbl[], "# found"=w757:i32)  [unwired: 3 in, 2 out]
                      n573 = call <vilib>:"Peak Detector.vi"("peaks/valleys"=enum32{"Peaks", "Valleys"}."Valleys", "width"=w754, "threshold"=w730, "X"=w729) -> ("Amplitudes"=w755:dbl[], "Locations"=w752:dbl[])  [unwired: 3 in, 3 out]
                      n574 = Less Than 0?(x=w756) -> (x < 0?=w758:bool[])
                      n575 = Less Than 0?(x=w755) -> (x < 0?=w760:bool[])
                      n576 = Boolean To (0,1)(Boolean=w758) -> (0, 1=w768:i16[])
                      n577 = Boolean To (0,1)(Boolean=w760) -> (0, 1=w761:i16[])
                      n578 = To Double Precision Float(number=w768) -> (double precision float=w759:dbl[])
                      n579 = To Double Precision Float(number=w761) -> (double precision float=w762:dbl[])
                      n580 = Build Array(w753, w759) -> (w764:dbl[][])
                      n581 = Build Array(w752, w762) -> (w763:dbl[][])
                      n582 = Insert Into Array(array=w764, index (col)=w757, new element=w763) -> (w765:dbl[][])  [unwired: 1 in]
                      n583 = call "Sort 2D Array.vim"("index"=0, "dimension to index (column)"=enum16{"column", "row"}."row", "2D array"=w765) -> ("sorted 2D array"=w743:dbl[][])  [unwired: 7 in, 1 out]
                      n584 = Index Array(array=w743) -> (element #1=w739:dbl[], element #2=w742:dbl[])  [unwired: 4 in]
                      n585 = Multiply(x=w739, y=w738) -> (x*y=w737:dbl[])
                      n586 = Equal?(x=w742, y=w735) -> (x = y?=w751:bool[])
                      n587 = Boolean Array To Number(Boolean array=w751) -> (number=w750:u32)
                      n588 = Array Size(array=w735) -> (size(s)=w747:i32)
                      n589 = To Double Precision Float(number=w747) -> (double precision float=w746:dbl)
                      n590 = Power Of X(1:2.0 ("x"), 2:w746) -> (0:w745:dbl)
                      n591 = Decrement(x=w745) -> (x-1=w749:dbl)
                      n592 = To Unsigned Long Integer(number=w749) -> (unsigned 32bit integer=w744:u32)
                      n593 = Equal?(x=w750, y=w744) -> (x = y?=w741:bool)
                      n594 = case shown="참" w741 {
                        tunnel: w737 -> [_ w776]
                        tunnel: dbl[] [inf, inf, inf, inf, inf, inf, inf, inf] -> [w773 w775]
                        tunnel: [w773 w774] -> w736
                        frame False {
                        }
                        frame True {
                          n595 = Replace Array Subset(array=w775, new element=w776) -> (w774:dbl[])  [unwired: 1 in]
                        }
                      }
                    }
                  }
                  n596 = flat-sequence {
                    tunnel: w523 -> [w627]
                    tunnel: w522 -> [w625]
                    tunnel: w521 -> [w624]
                    tunnel: w524 -> [w622]
                    tunnel: w520 -> [w620]
                    tunnel: [w621] -> w528
                    tunnel: [w620] -> w527
                    tunnel: w518 -> [w619]
                    tunnel: [w619] -> w526
                    tunnel: w519 -> [w618]
                    tunnel: [w618] -> w525
                    tunnel: w502 -> [w617]
                    tunnel: [w617] -> w501
                    tunnel: w528 -> [w654]
                    tunnel: w527 -> [w691]
                    tunnel: w526 -> [w658]
                    tunnel: [w656] -> w510
                    tunnel: w525 -> [w655]
                    tunnel: w501 -> [w651]
                    frame #0 {
                      n597 = Obtain Queue(name (unnamed)="ch7" ("이름(이름없음)"), element data type=w627) -> (queue out=w631:refnum<queue>, error out=w630:errorcluster)  [unwired: 3 in, 1 out]
                      n598 = for {
                        N: w622 -> [_]
                        tunnel: w631 -> [w648]
                        tunnel: w630 -> [w647]
                        tunnel: [w646] -> w629
                        tunnel: [w645] -> w628
                        tunnel: w625 -> [w635]
                        tunnel: w624 -> [w634]
                        tunnel: [w632] -> w623 mode=indexing
                        w633 = TRUE ("init/cont (init:F)")
                        n599 = Dequeue Element(queue=w648, error in (no error)=w647) -> (queue out=w646:refnum<queue>, element=w640:waveform(dbl), error out=w645:errorcluster)  [unwired: 2 out]
                        n600 = Unbundle By Name(w640) -> ("Y"=w639:dbl[])
                        n601 = Unbundle By Name(w640) -> ("Y"=w638:dbl[])
                        n602 = call-poly <vilib>:"FIR Filter.vi"("init/cont (init:F)"=w633, "FIR Coefficients"=w635, "X"=w639) -> ("Filtered X"=w644:dbl[])  [unwired: 1 in, 1 out]
                        n603 = call-poly <vilib>:"FIR Filter.vi"("init/cont (init:F)"=w633, "FIR Coefficients"=w634, "X"=w638) -> ("Filtered X"=w643:dbl[])  [unwired: 1 in, 1 out]
                        n604 = call "Envelope(SubVI).vi"("x"=w644) -> ("Y"=w642:dbl[])
                        n605 = call "Envelope(SubVI).vi"("x"=w643) -> ("Y"=w641:dbl[])
                        n606 = Square(x=w642) -> (x^2=w637:dbl[])
                        n607 = Square(x=w641) -> (x^2=w636:dbl[])
                        n608 = Subtract(x=w637, y=w636) -> (x-y=w632:dbl[])
                      }
                      n609 = Release Queue(queue=w629, error in (no error)=w628) -> ()  [unwired: 1 in, 3 out]
                      n610 = call "2Dto1D(SubVI).vi"("X1"=w623) -> ("Y1"=w621:dbl[])
                    }
                    frame #1 {
                      w674 = 75 ("width")
                      # "Sort"
                      # "Decision"
                      n611 = call-poly <vilib>:"FIR Filter.vi"("FIR Coefficients"=w691, "X"=w654) -> ("Filtered X"=w692:dbl[])  [unwired: 2 in, 1 out]
                      n612 = Array Max & Min(array=w692) -> (max value=w653:dbl, min value=w652:dbl)  [unwired: 2 out]
                      n613 = Add(x=w651, y=w653) -> (x+y=w650:dbl)
                      n614 = Subtract(x=w652, y=w651) -> (x-y=w649:dbl)
                      n615 = call <vilib>:"Peak Detector.vi"("peaks/valleys"=enum32{"Peaks", "Valleys"}."Peaks", "width"=w674, "threshold"=w650, "X"=w654) -> ("Amplitudes"=w676:dbl[], "Locations"=w673:dbl[], "# found"=w677:i32)  [unwired: 3 in, 2 out]
                      n616 = call <vilib>:"Peak Detector.vi"("peaks/valleys"=enum32{"Peaks", "Valleys"}."Valleys", "width"=w674, "threshold"=w649, "X"=w654) -> ("Amplitudes"=w675:dbl[], "Locations"=w672:dbl[])  [unwired: 3 in, 3 out]
                      n617 = Less Than 0?(x=w676) -> (x < 0?=w678:bool[])
                      n618 = Less Than 0?(x=w675) -> (x < 0?=w680:bool[])
                      n619 = Boolean To (0,1)(Boolean=w678) -> (0, 1=w688:i16[])
                      n620 = Boolean To (0,1)(Boolean=w680) -> (0, 1=w681:i16[])
                      n621 = To Double Precision Float(number=w688) -> (double precision float=w679:dbl[])
                      n622 = To Double Precision Float(number=w681) -> (double precision float=w682:dbl[])
                      n623 = Build Array(w673, w679) -> (w684:dbl[][])
                      n624 = Build Array(w672, w682) -> (w683:dbl[][])
                      n625 = Insert Into Array(array=w684, index (col)=w677, new element=w683) -> (w685:dbl[][])  [unwired: 1 in]
                      n626 = call "Sort 2D Array.vim"("index"=0, "dimension to index (column)"=enum16{"column", "row"}."row", "2D array"=w685) -> ("sorted 2D array"=w663:dbl[][])  [unwired: 7 in, 1 out]
                      n627 = Index Array(array=w663) -> (element #1=w659:dbl[], element #2=w662:dbl[])  [unwired: 4 in]
                      n628 = Multiply(x=w659, y=w658) -> (x*y=w657:dbl[])
                      n629 = Equal?(x=w662, y=w655) -> (x = y?=w671:bool[])
                      n630 = Boolean Array To Number(Boolean array=w671) -> (number=w670:u32)
                      n631 = Array Size(array=w655) -> (size(s)=w667:i32)
                      n632 = To Double Precision Float(number=w667) -> (double precision float=w666:dbl)
                      n633 = Power Of X(1:2.0 ("x"), 2:w666) -> (0:w665:dbl)
                      n634 = Decrement(x=w665) -> (x-1=w669:dbl)
                      n635 = To Unsigned Long Integer(number=w669) -> (unsigned 32bit integer=w664:u32)
                      n636 = Equal?(x=w670, y=w664) -> (x = y?=w661:bool)
                      n637 = case shown="참" w661 {
                        tunnel: w657 -> [_ w696]
                        tunnel: dbl[] [inf, inf, inf, inf, inf, inf, inf, inf] -> [w693 w695]
                        tunnel: [w693 w694] -> w656
                        frame False {
                        }
                        frame True {
                          n638 = Replace Array Subset(array=w695, new element=w696) -> (w694:dbl[])  [unwired: 1 in]
                        }
                      }
                    }
                  }
                }
                frame #1 {
                  w1318 = dbl[] []
                  # "First sensor"
                  # "If code detected,"
                  n639 = Add Array Elements(numeric array=w1317) -> (sum=w1328:dbl)
                  n640 = Add Array Elements(numeric array=w1316) -> (sum=w1327:dbl)
                  n641 = Add Array Elements(numeric array=w1315) -> (sum=w1326:dbl)
                  n642 = Add Array Elements(numeric array=w1314) -> (sum=w1325:dbl)
                  n643 = Add Array Elements(numeric array=w1313) -> (sum=w1324:dbl)
                  n644 = Add Array Elements(numeric array=w1312) -> (sum=w1323:dbl)
                  n645 = Add Array Elements(numeric array=w1311) -> (sum=w1322:dbl)
                  n646 = Add Array Elements(numeric array=w1310) -> (sum=w1321:dbl)
                  n647 = Insert Into Array(array=w1318, new element #1=w1328, new element #2=w1327, new element #3=w1326, new element #4=w1325, new element #5=w1324, new element #6=w1323, new element #7=w1322, new element #8=w1321) -> (w1320:dbl[])  [unwired: 1 in]
                  n648 = Array Max & Min(array=w1320) -> (min value=w1309:dbl, min index (indices)=w1319:i32)  [unwired: 2 out]
                  n649 = Less?(x=w1309, y=inf) -> (x < y?=w1308:bool)
                  n650 = case shown="참" w1308 {
                    tunnel: w1320 -> [_ w1374]
                    tunnel: [-1.0 w1361] -> w1304
                    tunnel: w1319 -> [_ w1360]
                    tunnel: w1309 -> [_ w1350]
                    tunnel: w1318 -> [_ w1349]
                    tunnel: w1317 -> [_ w1348]
                    tunnel: w1316 -> [_ w1347]
                    tunnel: w1315 -> [_ w1346]
                    tunnel: w1314 -> [_ w1345]
                    tunnel: w1313 -> [_ w1344]
                    tunnel: w1312 -> [_ w1343]
                    tunnel: w1311 -> [_ w1342]
                    tunnel: w1310 -> [_ w1341]
                    tunnel: [-1.0 w1334] -> w1303
                    tunnel: w1306 -> [w1330 _]
                    tunnel: [w1329 0] -> w1305
                    frame False {
                      n651 = Increment(x=w1330) -> (x+1=w1329:i32)
                    }
                    frame True {
                      w1351 = 1500.0
                      # "Sensor spacing : 39mm"
                      # "Sound speed : 1500m/s"
                      # "Check\nclockwise/counterclockwise\ndirection"
                      # "Confirmation of adjacent sensor extraction"
                      # "Second sensor sensor"
                      n652 = local read "Symbol length(sec)"() -> (w1338:dbl)
                      n653 = Insert Into Array(array=w1349, new element #1=w1348, new element #2=w1347, new element #3=w1346, new element #4=w1345, new element #5=w1344, new element #6=w1343, new element #7=w1342, new element #8=w1341) -> (w1340:dbl[])  [unwired: 1 in]
                      n654 = Array Max & Min(array=w1340) -> (min value=w1339:dbl)  [unwired: 3 out]
                      n655 = Replace Array Subset(array=w1374, new element=inf ("새 원소/부분배열"), index=w1360) -> (w1372:dbl[])
                      n656 = Subtract(x=w1339, y=w1338) -> (x-y=w1337:dbl)
                      n657 = Array Max & Min(array=w1372) -> (min value=w1364:dbl, min index (indices)=w1358:i32)  [unwired: 2 out]
                      n658 = Divide(x=w1351, y=0.039) -> (x/y=w1362:dbl)
                      n659 = Multiply(x=w1351, y=w1337) -> (x*y=w1336:dbl)
                      n660 = Divide(x=w1336, y=2.0) -> (x/y=w1334:dbl)
                      n661 = Subtract(x=w1360, y=w1358) -> (x-y=w1366:i32)
                      n662 = Equal?(x=w1360, y=0) -> (x = y?=w1356:bool)
                      n663 = Equal?(x=w1358, y=7) -> (x = y?=w1355:bool)
                      n664 = Absolute Value(x=w1366) -> (abs(x)=w1365:i32)
                      n665 = Greater?(x=w1360, y=w1358) -> (0:w1354:bool)
                      n666 = And(x=w1356, y=w1355) -> (x .and. y?=w1353:bool)
                      n667 = Equal?(x=w1365, y=1) -> (x = y?=w1369:bool)
                      n668 = Equal?(x=w1365, y=7) -> (x = y?=w1368:bool)
                      n669 = Or(x=w1354, y=w1353) -> (x .or. y?=w1352:bool)
                      n670 = Or(x=w1369, y=w1368) -> (x .or. y?=w1367:bool)
                      n671 = case shown="참" w1367 {
                        tunnel: w1352 -> [_ w1397]
                        tunnel: w1364 -> [_ w1396]
                        tunnel: w1350 -> [_ w1395]
                        tunnel: w1362 -> [_ w1394]
                        tunnel: w1360 -> [w1376 w1381]
                        tunnel: [w1375 w1379] -> w1361
                        frame False {
                          # "If two adjacent sensors are not extracted,\nEstimated in the direction of the sensor with the fastest arrival time"
                          n672 = To Double Precision Float(number=w1376) -> (double precision float=w1378:dbl)
                          n673 = Multiply(x=w1378, y=45.0) -> (x*y=w1375:dbl)
                        }
                        frame True {
                          # "DoA estimation"
                          # "Average of the difference\nover 8 bits of arrival time"
                          # "If two adjacent sensors are extracted,"
                          n674 = Subtract(x=w1396, y=w1395) -> (x-y=w1399:dbl)
                          n675 = Divide(x=w1399, y=8.0) -> (x/y=w1393:dbl)
                          n676 = Multiply(x=w1393, y=w1394) -> (x*y=w1392:dbl)
                          n677 = Inverse Cosine(1:w1392) -> (0:w1388:dbl)
                          n678 = Divide(x=180.0, y=3.141592653589793) -> (x/y=w1391:dbl)
                          n679 = Multiply(x=w1388, y=w1391) -> (x*y=w1382:dbl)
                          n680 = To Double Precision Float(number=w1381) -> (double precision float=w1384:dbl)
                          n681 = Subtract(x=w1382, y=67.5) -> (x-y=w1386:dbl)
                          n682 = Multiply(x=w1384, y=45.0) -> (x*y=w1387:dbl)
                          n683 = Add(x=w1386, y=w1387) -> (x+y=w1380:dbl)
                          n684 = case shown="거짓" w1397 {
                            tunnel: w1380 -> [w1400 w1402]
                            tunnel: [w1400 w1401] -> w1379
                            frame False {
                              # "Counter\nclockwise"
                            }
                            frame True {
                              # "clockwise"
                              n685 = Subtract(x=360.0 ("y"), y=w1402) -> (x-y=w1401:dbl)
                            }
                          }
                        }
                      }
                    }
                  }
                  "Signal processing" <- TRUE
                }
                frame #2 {
                  w1405 = waveform(dbl) {"t0"=timestamp(0 s since 1904-01-01), "dt"=1.0, "Y"=[]} ("Waveform")
                  w1461 = "AIzaSyCRJTyXL0g6x8KOfjPVXr0B6P1-pqc0a54"  # Google Maps API Key
                  # "Queue clear"
                  n686 = Number To Decimal String(number="Zoom") -> (decimal integer string=w1476:string)  [unwired: 1 in]
                  n687 = Number To Decimal String(number="Size Y") -> (decimal integer string=w1478:string)  [unwired: 1 in]
                  n688 = Number To Decimal String(number="Size X") -> (decimal integer string=w1480:string)  [unwired: 1 in]
                  n689 = Unbundle By Name(T2 {"Marker"="", "Path"="", "Markers Coordinates"=[]}) -> ("Marker"=w1464:string, "Path"=w1463:string)
                  n690 = Concatenate Strings("https://maps.googleapis.com/maps/api/staticmap?center=" ("URL"), "Latitude", "," ("string"), "Logitude", "&zoom=", w1476, "&size=", w1478, "x", w1480, "&maptype=", "Map Format") -> (w1465:string)
                  n691 = Concatenate Strings(w1465, w1464, w1463, "&key=" ("string"), w1461) -> (w1453:string)
                  n692 = flat-sequence {
                    tunnel: w1453 -> [w1485]
                    tunnel: [w1482] -> w1452
                    frame #0 {
                      n693 = call <vilib>:"OpenHandle.vi"() -> ("client handle out"=w1489:T3, "error out"=w1488:errorcluster)  [unwired: 14 in]
                      n694 = Temporary Directory() -> (w1483:path)
                      n695 = Build Path(base path=w1483, name or relative path="map.png") -> (appended path=w1482:path)
                      n696 = call <vilib>:"GET.vi"("client handle"=w1489, "output file"=w1482, "url"=w1485, "error in (no error)"=w1488) -> ("client handle out"=w1486:T3, "error out"=w1487:errorcluster)  [unwired: 8 in, 2 out]
                      n697 = call <vilib>:"CloseHandle.vi"("client handle"=w1486, "error in (no error)"=w1487) -> ()  [unwired: 13 in, 1 out]
                    }
                  }
                  n698 = for {
                    N: 1 -> [_]
                    tunnel: [w1492] -> w1457 mode=indexing
                    tunnel: w1448 -> [w1491]
                    tunnel: w1447 -> [w1490]
                    n699 = Bundle(w1490, w1491) -> (w1492:cluster{dbl, dbl})  [unwired: 1 in]
                  }
                  n700 = invoke class="IWebBrowser2" method="Navigate"(reference="WebBrowser", "URL"=w1453) -> ()  [unwired: 6 in, 8 out]
                  n701 = call <vilib>:"Read PNG File.vi"("path to PNG file"=w1452) -> ("image data"=w1451:T4)  [unwired: 8 in, 2 out]
                  n702 = call <vilib>:"Draw Flattened Pixmap.vi"("image data"=w1451) -> ("new picture"=w1450:picture)  [unwired: 1 in, 7 out]
                  n703 = property on="Scope" class="Pict"() -> ("Draw Area Size"=w1458:T5)  [unwired: 2 in, 2 out]
                  n704 = call <vilib>:"Polar Plot with Point Options.vi"("picture"=w1450, "data array [mag, phase (deg)]"=w1457, "dimensions (w,h)"=w1458, "polar attributes"=T1 {"maximum"=1500.0, "minimum"=0.0, "clip to min"=FALSE, "log?(F)"=FALSE, "grid color"=15718400, "plot color"=13107268, "fmt and prec"={"format"=enum."Decimal", "precision"=2}, "visible section"=8}, "Lines/Points"=enum16{"Lines", "Points"}."Points", "Size"=u16 15) -> ("new picture"=→"Scope":picture)  [unwired: 9 in]
                  n705 = Obtain Queue(name (unnamed)="ch1" ("이름(이름없음)"), element data type=w1405) -> (queue out=w1437:refnum<queue>, error out=w1436:errorcluster)  [unwired: 3 in, 1 out]
                  n706 = Obtain Queue(name (unnamed)="ch3" ("이름(이름없음)"), element data type=w1405) -> (queue out=w1428:refnum<queue>, error out=w1427:errorcluster)  [unwired: 3 in, 1 out]
                  n707 = Obtain Queue(name (unnamed)="ch4" ("이름(이름없음)"), element data type=w1405) -> (queue out=w1423:refnum<queue>, error out=w1422:errorcluster)  [unwired: 3 in, 1 out]
                  n708 = Obtain Queue(name (unnamed)="ch6" ("이름(이름없음)"), element data type=w1405) -> (queue out=w1414:refnum<queue>, error out=w1413:errorcluster)  [unwired: 3 in, 1 out]
                  n709 = Obtain Queue(name (unnamed)="ch7" ("이름(이름없음)"), element data type=w1405) -> (queue out=w1407:refnum<queue>, error out=w1406:errorcluster)  [unwired: 3 in, 1 out]
                  n710 = Obtain Queue(name (unnamed)="ch0" ("이름(이름없음)"), element data type=w1405) -> (queue out=w1445:refnum<queue>, error out=w1444:errorcluster)  [unwired: 3 in, 1 out]
                  n711 = Obtain Queue(name (unnamed)="ch2" ("이름(이름없음)"), element data type=w1405) -> (queue out=w1435:refnum<queue>, error out=w1434:errorcluster)  [unwired: 3 in, 1 out]
                  n712 = Obtain Queue(name (unnamed)="ch5" ("이름(이름없음)"), element data type=w1405) -> (queue out=w1421:refnum<queue>, error out=w1420:errorcluster)  [unwired: 3 in, 1 out]
                  n713 = Flush Queue(queue=w1445, error in (no error)=w1444) -> (queue out=w1443:refnum<queue>, error out=w1442:errorcluster)  [unwired: 1 out]
                  n714 = Flush Queue(queue=w1437, error in (no error)=w1436) -> (queue out=w1439:refnum<queue>, error out=w1438:errorcluster)  [unwired: 1 out]
                  n715 = Flush Queue(queue=w1435, error in (no error)=w1434) -> (queue out=w1433:refnum<queue>, error out=w1432:errorcluster)  [unwired: 1 out]
                  n716 = Flush Queue(queue=w1428, error in (no error)=w1427) -> (queue out=w1430:refnum<queue>, error out=w1429:errorcluster)  [unwired: 1 out]
                  n717 = Flush Queue(queue=w1423, error in (no error)=w1422) -> (queue out=w1425:refnum<queue>, error out=w1424:errorcluster)  [unwired: 1 out]
                  n718 = Flush Queue(queue=w1421, error in (no error)=w1420) -> (queue out=w1419:refnum<queue>, error out=w1418:errorcluster)  [unwired: 1 out]
                  n719 = Flush Queue(queue=w1414, error in (no error)=w1413) -> (queue out=w1416:refnum<queue>, error out=w1415:errorcluster)  [unwired: 1 out]
                  n720 = Flush Queue(queue=w1407, error in (no error)=w1406) -> (queue out=w1409:refnum<queue>, error out=w1408:errorcluster)  [unwired: 1 out]
                  n721 = Release Queue(queue=w1443, error in (no error)=w1442) -> ()  [unwired: 1 in, 3 out]
                  n722 = Release Queue(queue=w1439, error in (no error)=w1438) -> ()  [unwired: 1 in, 3 out]
                  n723 = Release Queue(queue=w1433, error in (no error)=w1432) -> ()  [unwired: 1 in, 3 out]
                  n724 = Release Queue(queue=w1430, error in (no error)=w1429) -> ()  [unwired: 1 in, 3 out]
                  n725 = Release Queue(queue=w1425, error in (no error)=w1424) -> ()  [unwired: 1 in, 3 out]
                  n726 = Release Queue(queue=w1419, error in (no error)=w1418) -> ()  [unwired: 1 in, 3 out]
                  n727 = Release Queue(queue=w1416, error in (no error)=w1415) -> ()  [unwired: 1 in, 3 out]
                  n728 = Release Queue(queue=w1409, error in (no error)=w1408) -> ()  [unwired: 1 in, 3 out]
                  "DoA" <- w1448
                  "Distance" <- w1447
                  "DoA Estimation" <- TRUE ("DoA Estimation")
                  "not detected number" <- w1404
                }
                frame #3 {
                  "Display" <- TRUE ("Display")
                }
              }
              n729 = Greater Or Equal?(x=w488, y=5) -> (x >= y?=w486:bool)
              "DoA trial number" <- w481
            }
          }
        }
      }
    }
  }
